vi "Test_Multiple Class_Multiple State.vi"() -> ()   [LabVIEW 2021]
uses:
  Commander/Commander.lvclass
  C:/Program Files (x86)/Hyper State Machine Framework/SSW_Hyper_State_Machine.lvlibp/State_Machine_Class/Main_State_Machine/Hyper_State_Machine.lvclass
  C:/Program Files (x86)/Hyper State Machine Framework/SSW_Hyper_State_Machine.lvlibp/State_Interface/State_Interface.lvclass
  Common_State/Common_State.lvclass
  Image_Acquisition/Image_Acquisition.lvclass
  Motion_Control/Motion_Control.lvclass
  Data_Logging/Data_Logging.lvclass
  DIO/DIO.lvclass
  C:/Program Files (x86)/Hyper State Machine Framework/SSW_Hyper_State_Machine.lvlibp/State_Machine_Class/State_Machine_Module.llb/State Machine.ctl
  C:/Program Files (x86)/Hyper State Machine Framework/SSW_Hyper_State_Machine.lvlibp/State_Machine_Class/State_Machine_Module.llb/Lock_Unlock.ctl
  C:/Program Files (x86)/Hyper State Machine Framework/SSW_Hyper_State_Machine.lvlibp/State_Machine_Class/State_Machine_Module.llb/Iterval.ctl
  C:/Program Files (x86)/Hyper State Machine Framework/SSW_Hyper_State_Machine.lvlibp/State_Machine_Class/State_Machine_Module.llb/Time_Out.ctl
  <vilib>/numeric/Random Number (Range) DBL.vi
  <vilib>/Utility/High Resolution Relative Seconds.vi
  C:/Program Files (x86)/Hyper State Machine Framework/SSW_Hyper_State_Machine.lvlibp
panel:
  out "Activate":bool
  out "Lamp":bool
  out "Current_Pos":dbl caption="mm"
  in  "EMO":bool
  out "Product ID":string
  in  "Activate_Code(Blank for 30 min Trial)":string="ROeInPkJ3DxAXwEgzbbW2XA0t1jaS1URlS9jikesQMED6VfU"
  out "Heart_Rate":bool
  out "Heart rate(s)":dbl format="%#_6p"
  out "Execute rate(Hz)":dbl format="%#_6p"
  out "Base Class_Time_Act":bool
  out "Base Class_Elapsed Time(s)":dbl format="%#_6p"
  out "Base Class":bool=TRUE
  out "Base Class_Remaining(s)":dbl format="%#_6p"
  out "Base Class Progress":dbl(slide) scale=0.0..10.0
  in  "Base Class":dbl=10.0 max=1000.0 format="%#_13p"
  out "Base Class":string
  out "Base Class_Active":bool
  in  "Action Manager":T1(ring)
  out "Common":bool=TRUE
  out "Common_State":string
  out "Common_Time_Act":bool
  out "Common_Elapsed Time(s)":dbl format="%#_6p"
  out "Common_State Progress":dbl(slide) scale=0.0..5.0
  in  "Common_State_Interval":dbl=5.0 max=1000.0 format="%#_13p"
  out "Common_State_Active":bool
  out "Common_State_Remaining(s)":dbl format="%#_6p"
  out "Data Logging Progress":dbl(slide) scale=0.0..3.0
  out "DIO Progress":dbl(slide) scale=0.0..0.01
  out "Motion Control Progress":dbl(slide) scale=0.0..0.5
  out "Image Acquisition Progress":dbl(slide) scale=0.0..0.25
  out "Commander Progress":dbl(slide)=-1.0 scale=0.0..1.0
  out "Data_Logging":bool=TRUE
  out "Data Logging":string
  out "Data_Logging_Time_Act":bool
  out "Data_Logging_Elapsed Time(s)":dbl format="%#_6p"
  out "DIO":bool=TRUE
  out "DIO":string
  out "DIO_Time_Act":bool
  out "DIO_Elapsed Time(s)":dbl format="%#_6p"
  out "Motion_Control":bool=TRUE
  out "Motion_Control":string
  out "Motion_Control_Time_Act":bool
  out "Motion_Control_Elapsed Time(s)":dbl format="%#_6p"
  in  "Data Logging":dbl=3.0 max=1000.0 format="%#_13p"
  out "Data Logging_Active":bool
  out "Data Logging_Remaining(s)":dbl format="%#_6p"
  in  "DIO_Interval":dbl=0.01 max=1000.0 format="%#_13p"
  in  "Motion_Control_Interval":dbl=0.5 max=1000.0 format="%#_13p"
  out "Motion Control_Act":bool
  out "DIO_Act":bool
  out "DIO_Remaining(s)":dbl format="%#_6p"
  out "Motion_Control_Remaining(s)":dbl format="%#_6p"
  in  "Image Acquisition_Interval":dbl=0.25 max=1000.0 format="%#_13p"
  in  "Commander_Interval":dbl max=1000.0 format="%#_13p"
  in  "System_Wait_Time":dbl=0.025 format="%#_13p"
  out "Commander_Active":bool
  out "Image Acquisition_Act":bool
  out "Image Acquisition_Remaining(s)":dbl format="%#_6p"
  out "Commander_Remaining(s)":dbl format="%#_6p"
  out "Image Acquisition":bool=TRUE
  out "Image Acquisition":string
  out "Commander":bool=TRUE
  out "Image Acquisition_Time_Act":bool
  out "Image Acquisition_Elapsed Time(s)":dbl format="%#_6p"
  out "Commander":string
  out "State1_Time_Act":bool
  out "Commander_Elapsed Time(s)":dbl format="%#_6p"
  in  "Stop":bool
  # "Note : Each State is Waiting Until Commader State Finished on \"Interval_Delay\" and then Unlock"
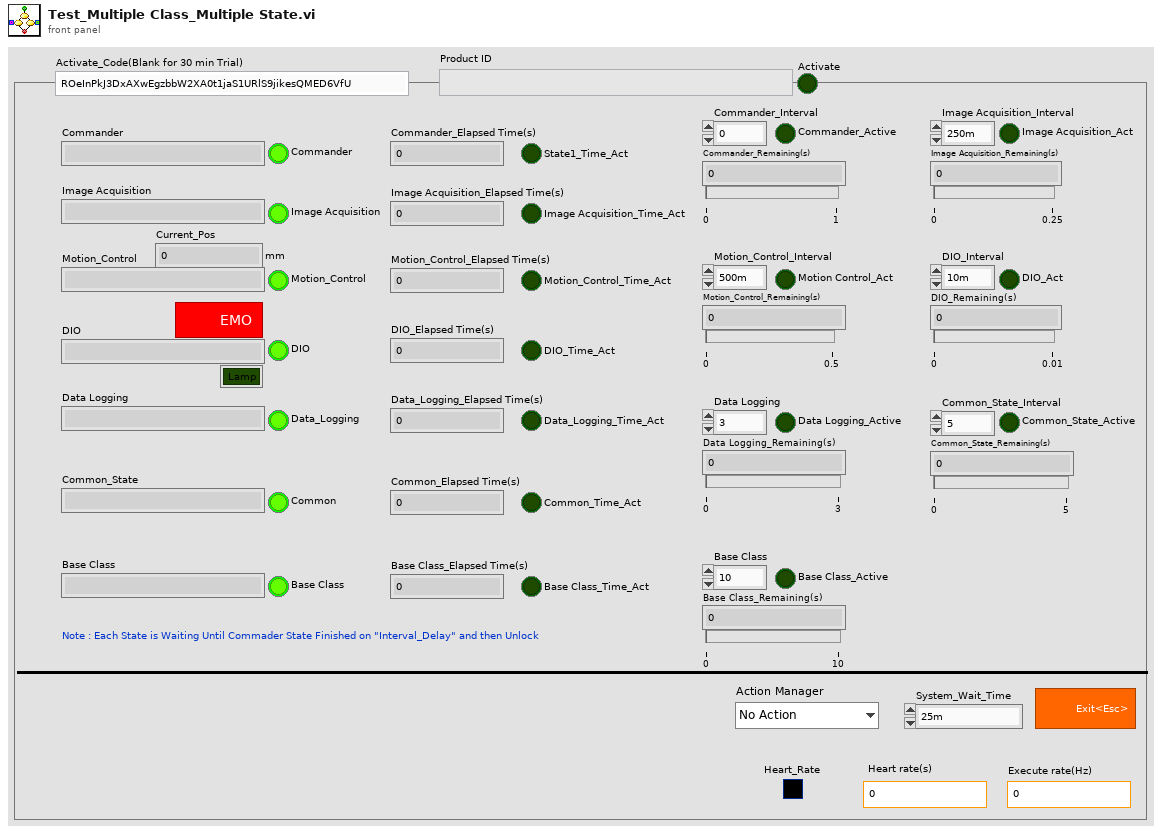
[diagram p1: front panel]
types:
  T1 = enum16{"No Action", "Init", "Lock", "Unlock", "Release"}
  T2 = typedef "SSW_Hyper_State_Machine.lvlibp/State Machine.ctl" = cluster{"Command":string, "Data":variant}
  T3 = typedef "SSW_Hyper_State_Machine.lvlibp/Time_Out.ctl" = cluster{"Enable(True)":bool, "Time Out_State Name":string, "Time Target (1s)":dbl, "Time Out_Reply Message_State":string}
  T4 = typedef "SSW_Hyper_State_Machine.lvlibp/Lock_Unlock.ctl" = cluster{"Action_Mode (Get)":enum16{"Set", "Get"}, "Action_Set (False)":bool, "State_In (Wait)":string}
  T5 = typedef "SSW_Hyper_State_Machine.lvlibp/Iterval.ctl" = cluster{"Delay(s)":dbl, "State (Interval_Delay)":string}
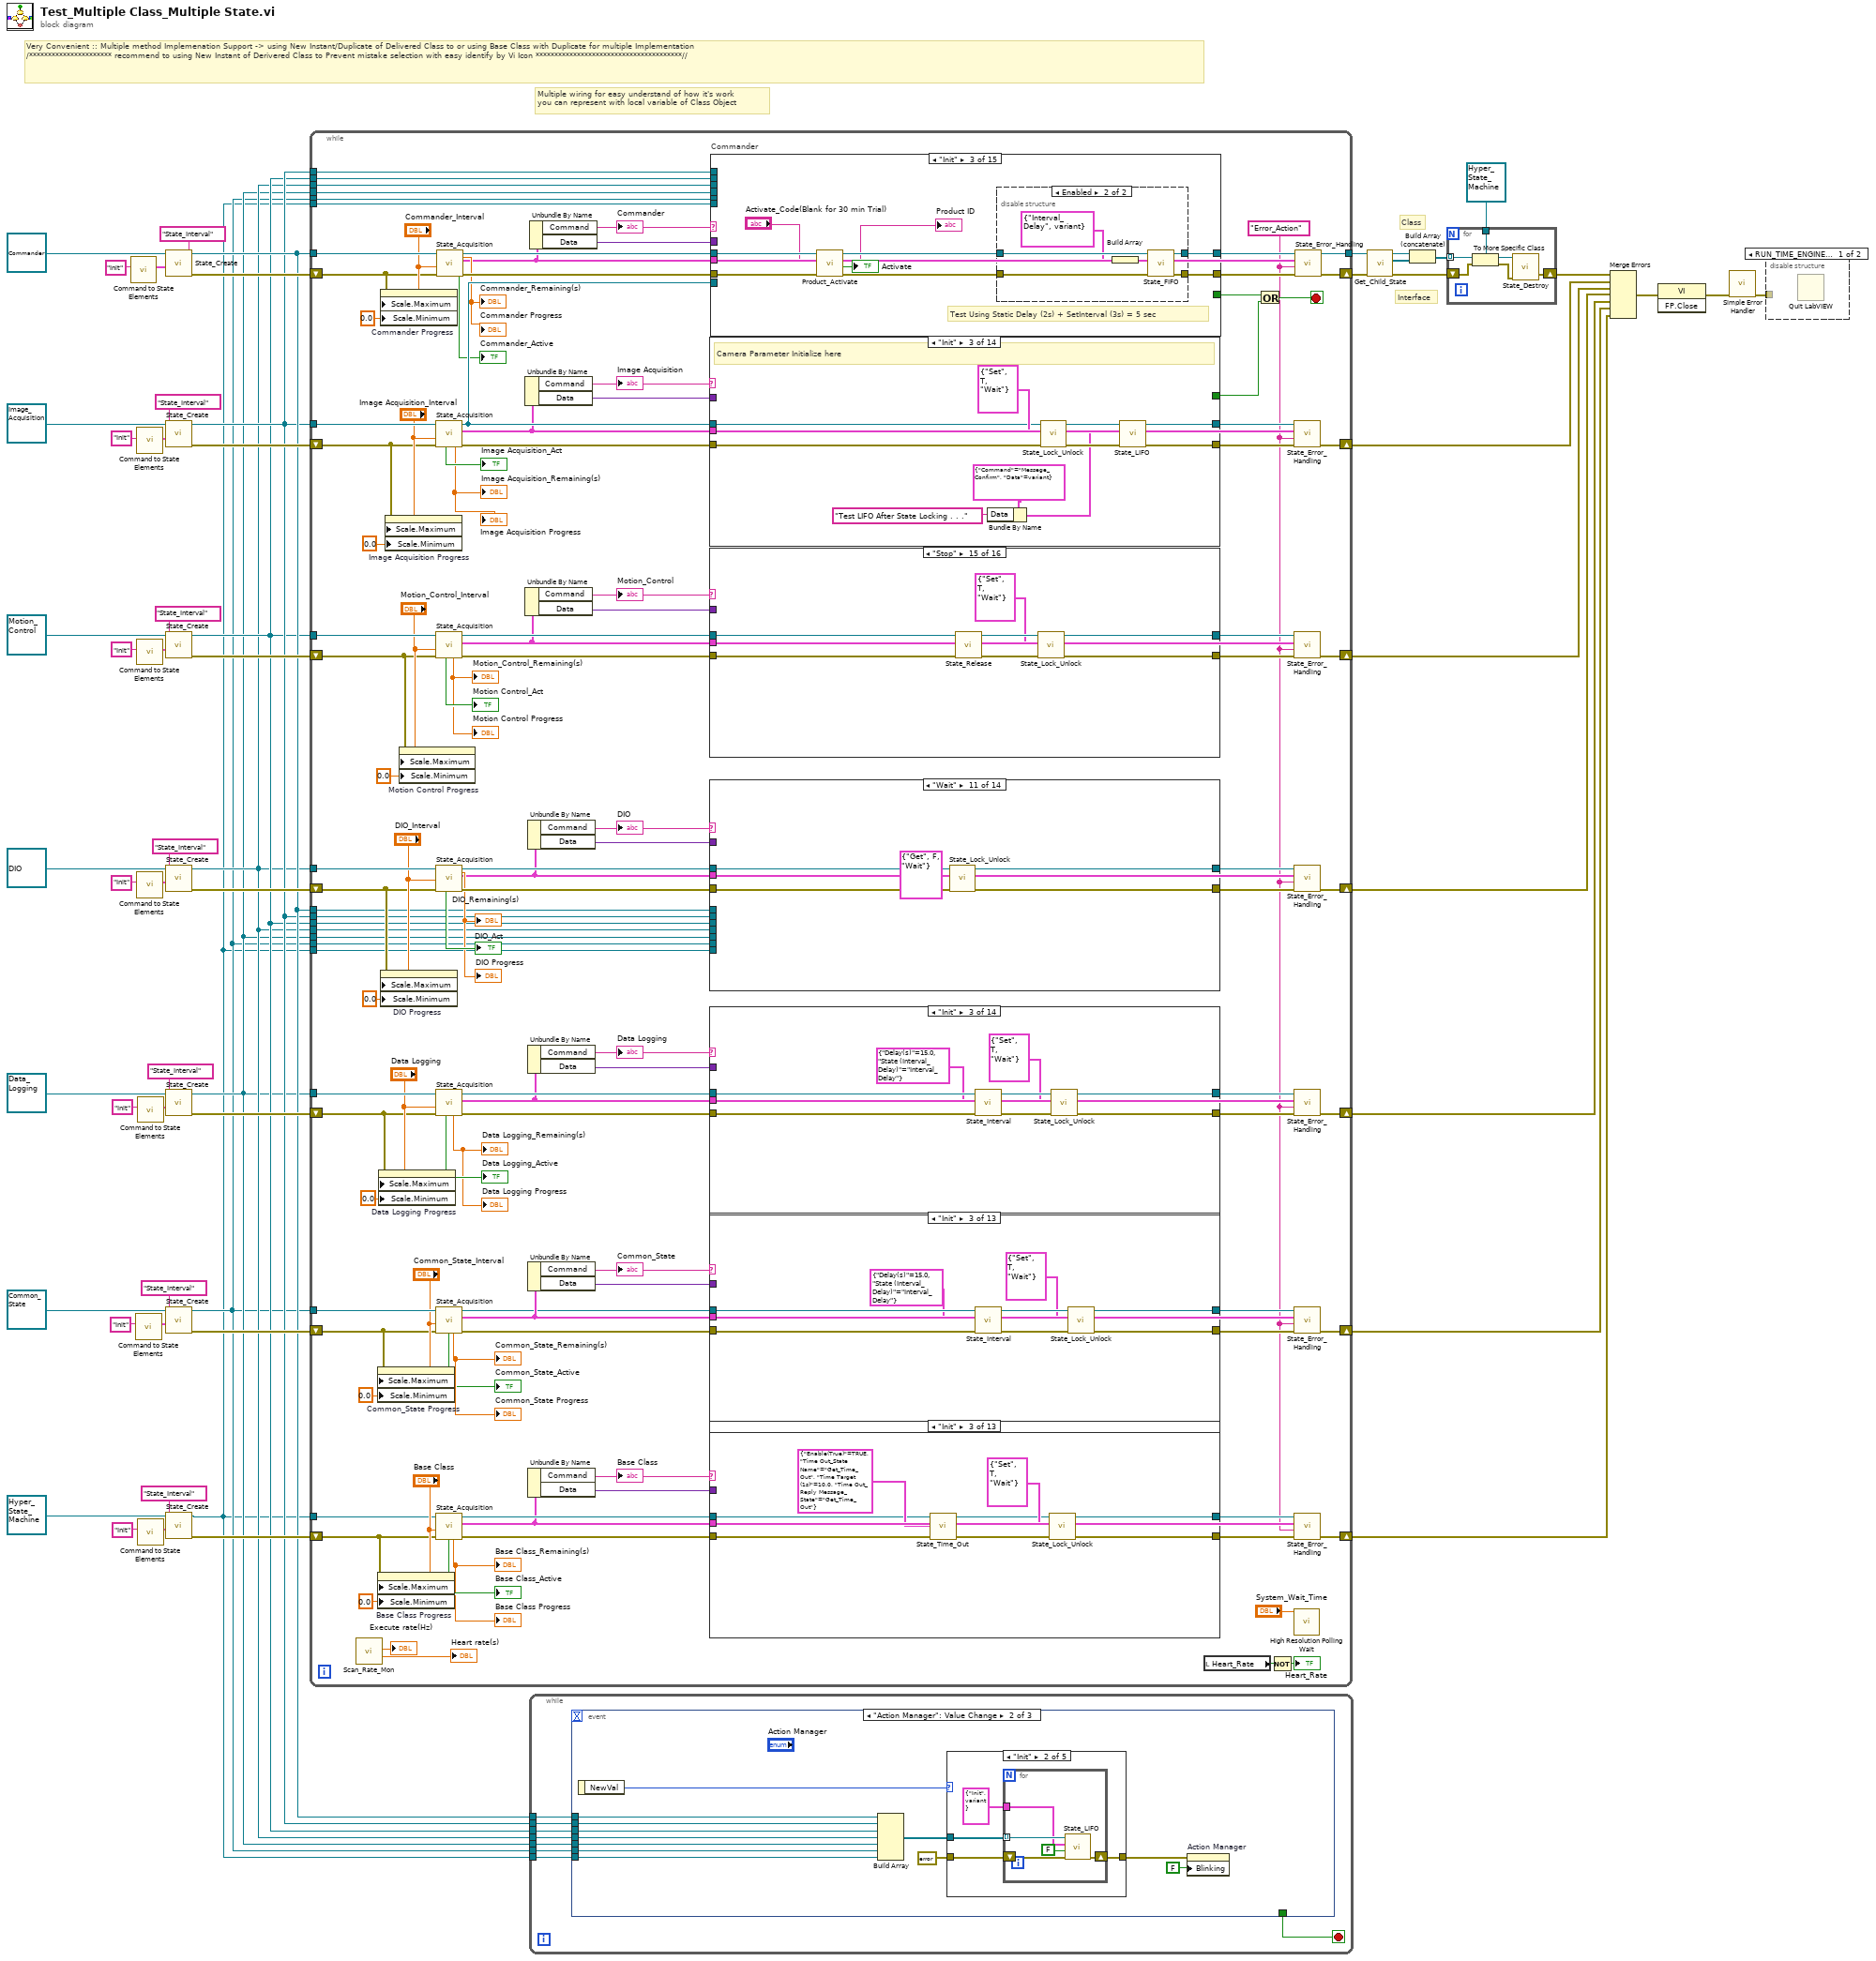
[diagram p0: block diagram]
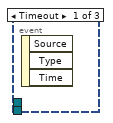
[diagram p3: hidden frame]
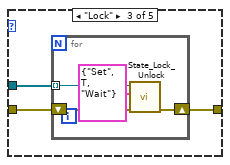
[diagram p5: hidden frame]
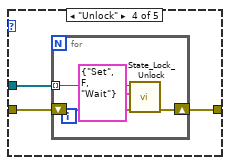
[diagram p6: hidden frame]
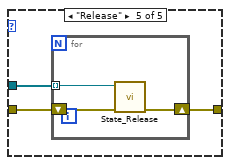
[diagram p7: hidden frame]
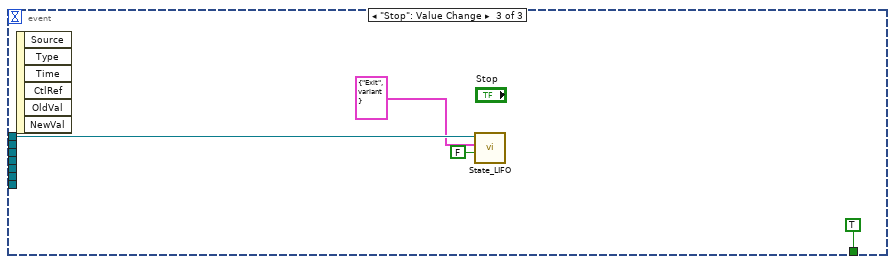
[diagram p8: hidden frame]
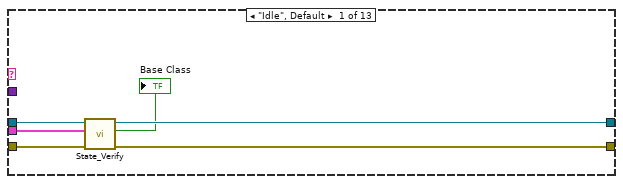
[diagram p9: hidden frame]
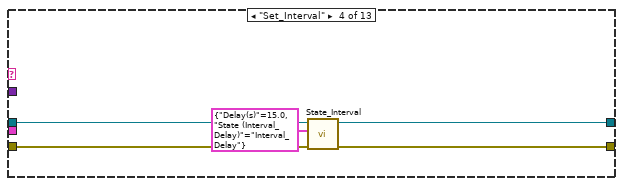
[diagram p11: hidden frame]
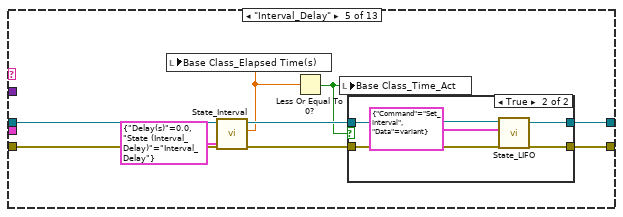
[diagram p12: hidden frame]
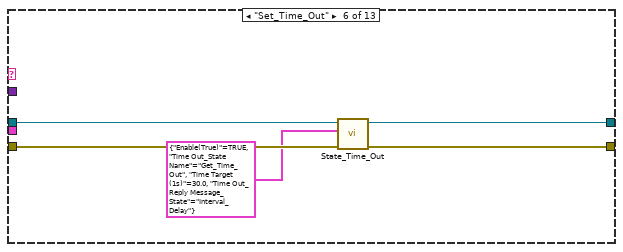
[diagram p14: hidden frame]
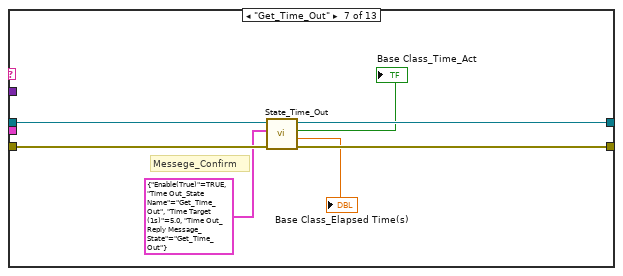
[diagram p15: hidden frame]
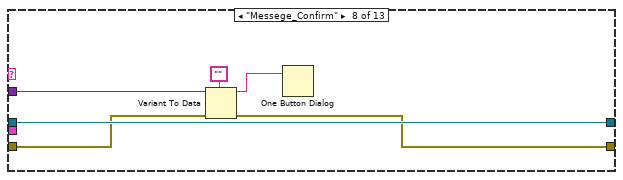
[diagram p16: hidden frame]
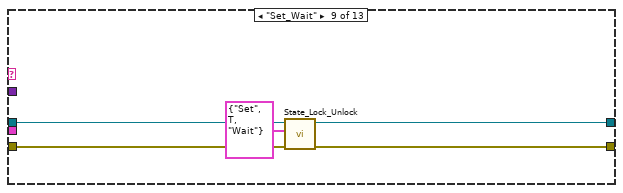
[diagram p17: hidden frame]
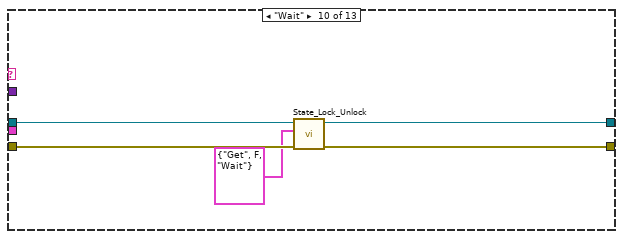
[diagram p18: hidden frame]
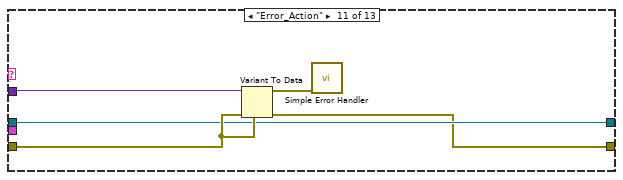
[diagram p19: hidden frame]
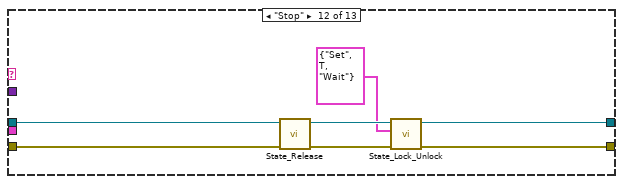
[diagram p20: hidden frame]
diagram:
  # "Interface"
  # "Class"
  # "Multiple wiring for easy understand of how it's work\nyou can represent with local variable of Class Object"
  # "Very Convenient :: Multiple method Implemenation Support -> using New Instant/Duplicate of Delivered Class to or using Base Class with Duplicate for multiple Implementation\n/********************** recommend to using New Instant of Derivered Class to Prevent mistake selection with easy identify by Vi Icon ***************************************//"
  n1 = call "Command to State Elements.vi"("Command"="Init") -> ("Command to State Elements"=w42:T2)  [unwired: 10 in]
  n2 = call "Command to State Elements.vi"("Command"="Init") -> ("Command to State Elements"=w34:T2)  [unwired: 10 in]
  n3 = call "Command to State Elements.vi"("Command"="Init") -> ("Command to State Elements"=w44:T2)  [unwired: 10 in]
  n4 = call "Command to State Elements.vi"("Command"="Init") -> ("Command to State Elements"=w40:T2)  [unwired: 10 in]
  n5 = call "Command to State Elements.vi"("Command"="Init") -> ("Command to State Elements"=w38:T2)  [unwired: 10 in]
  n6 = call "Command to State Elements.vi"("Command"="Init") -> ("Command to State Elements"=w36:T2)  [unwired: 10 in]
  n7 = call "Command to State Elements.vi"("Command"="Init") -> ("Command to State Elements"=w32:T2)  [unwired: 10 in]
  n8 = call-dynamic "State_Create.vi"("Init_State(Option)"=w42, "State_Interval_Name"="State_Interval" ("Core_Interval_Name(State_Interval)"), "State_Machine_Class in"=refnum<class "Commander.lvclass"> refnum ("Commander.lvclass")) -> ("error out"=w59:errorcluster, "State_Machine_Class out"=w24:refnum<class "Commander.lvclass">)  [unwired: 6 in, 1 out]
  n9 = call-dynamic "State_Create.vi"("Init_State(Option)"=w44, "State_Interval_Name"="State_Interval" ("Core_Interval_Name(State_Interval)"), "State_Machine_Class in"=refnum<class "Image_Acquisition.lvclass"> refnum ("Image_Acquisition.lvclass")) -> ("error out"=w58:errorcluster, "State_Machine_Class out"=w23:refnum<class "Image_Acquisition.lvclass">)  [unwired: 6 in, 1 out]
  n10 = call-dynamic "State_Create.vi"("Init_State(Option)"=w40, "State_Interval_Name"="State_Interval" ("Core_Interval_Name(State_Interval)"), "State_Machine_Class in"=refnum<class "Motion_Control.lvclass"> refnum ("Motion_Control.lvclass")) -> ("error out"=w53:errorcluster, "State_Machine_Class out"=w22:refnum<class "Motion_Control.lvclass">)  [unwired: 6 in, 1 out]
  n11 = call-dynamic "State_Create.vi"("Init_State(Option)"=w38, "State_Interval_Name"="State_Interval" ("Core_Interval_Name(State_Interval)"), "State_Machine_Class in"=refnum<class "DIO.lvclass"> refnum ("DIO.lvclass")) -> ("error out"=w52:errorcluster, "State_Machine_Class out"=w21:refnum<class "DIO.lvclass">)  [unwired: 6 in, 1 out]
  n12 = call-dynamic "State_Create.vi"("Init_State(Option)"=w36, "State_Interval_Name"="State_Interval" ("Core_Interval_Name(State_Interval)"), "State_Machine_Class in"=refnum<class "Data_Logging.lvclass"> refnum ("Data_Logging.lvclass")) -> ("error out"=w51:errorcluster, "State_Machine_Class out"=w20:refnum<class "Data_Logging.lvclass">)  [unwired: 6 in, 1 out]
  n13 = call-dynamic "State_Create.vi"("Init_State(Option)"=w34, "State_Interval_Name"="State_Interval" ("Core_Interval_Name(State_Interval)"), "State_Machine_Class in"=refnum<class "Common_State.lvclass"> refnum ("Common_State.lvclass")) -> ("error out"=w49:errorcluster, "State_Machine_Class out"=w19:refnum<class "Common_State.lvclass">)  [unwired: 6 in, 1 out]
  n14 = call-dynamic "State_Create.vi"("Init_State(Option)"=w32, "State_Interval_Name"="State_Interval" ("Core_Interval_Name(State_Interval)"), "State_Machine_Class in"=refnum<class "Hyper_State_Machine.lvclass"> refnum ("SSW_Hyper_State_Machine.lvlibp:Hyper_State_Machine.lvclass")) -> ("error out"=w46:errorcluster, "State_Machine_Class out"=w18:refnum<class "Hyper_State_Machine.lvclass">)  [unwired: 6 in, 1 out]
  n15 = while {
    tunnel: w24 -> [w166]
    shift-right: [w174] -> w16
    shift-left: w59 -> [w79]
    tunnel: [w173] -> w17
    tunnel: w23 -> [w169]
    shift-right: [w168] -> w9
    shift-left: w58 -> [w78]
    tunnel: w22 -> [w144]
    tunnel: w21 -> [w143]
    tunnel: w20 -> [w142]
    shift-right: [w141] -> w8
    shift-left: w53 -> [w77]
    shift-right: [w140] -> w7
    shift-left: w52 -> [w76]
    shift-right: [w139] -> w6
    shift-left: w51 -> [w75]
    tunnel: w19 -> [w118]
    shift-right: [w117] -> w5
    shift-left: w49 -> [w74]
    shift-right: [w87] -> w4
    shift-left: w46 -> [w73]
    tunnel: w18 -> [w91]
    tunnel: w23 -> [w72]
    tunnel: w22 -> [w71]
    tunnel: w21 -> [w70]
    tunnel: w20 -> [w69]
    tunnel: w19 -> [w68]
    tunnel: w18 -> [w67]
    tunnel: w24 -> [w66]
    tunnel: w23 -> [w65]
    tunnel: w22 -> [w64]
    tunnel: w21 -> [w63]
    tunnel: w20 -> [w62]
    tunnel: w19 -> [w61]
    tunnel: w18 -> [w60]
    stop <- w165 stop-if-true
    w86 = "Error_Action" ("State_Error_Handling")
    n16 = call "Scan_Rate_Mon.vi"() -> ("Heart rate(s)"=→"Heart rate(s)":dbl, "Execute rate(Hz)"=→"Execute rate(Hz)":dbl)
    n17 = property on="Common_State Progress" class="Slide (strict)"(error in=w74, "Scale.Maximum"="Common_State_Interval", "Scale.Minimum"=0.0 ("Scale.Range:Minimum")) -> ()  [unwired: 1 in, 2 out]
    n18 = property on="Base Class Progress" class="Slide (strict)"(error in=w73, "Scale.Maximum"="Base Class", "Scale.Minimum"=0.0 ("Scale.Range:Minimum")) -> ()  [unwired: 1 in, 2 out]
    n19 = property on="Data Logging Progress" class="Slide (strict)"(error in=w75, "Scale.Maximum"="Data Logging", "Scale.Minimum"=0.0 ("Scale.Range:Minimum")) -> ()  [unwired: 1 in, 2 out]
    n20 = property on="Commander Progress" class="Slide (strict)"(error in=w79, "Scale.Maximum"="Commander_Interval", "Scale.Minimum"=0.0 ("Scale.Range:Minimum")) -> ()  [unwired: 1 in, 2 out]
    n21 = property on="DIO Progress" class="Slide (strict)"(error in=w76, "Scale.Maximum"="DIO_Interval", "Scale.Minimum"=0.0 ("Scale.Range:Minimum")) -> ()  [unwired: 1 in, 2 out]
    n22 = property on="Image Acquisition Progress" class="Slide (strict)"(error in=w78, "Scale.Maximum"="Image Acquisition_Interval", "Scale.Minimum"=0.0 ("Scale.Range:Minimum")) -> ()  [unwired: 1 in, 2 out]
    n23 = property on="Motion Control Progress" class="Slide (strict)"(error in=w77, "Scale.Maximum"="Motion_Control_Interval", "Scale.Minimum"=0.0 ("Scale.Range:Minimum")) -> ()  [unwired: 1 in, 2 out]
    n24 = call-dynamic "State_Acquisition.vi"("error in (no error)"=w78, "State_Interval_Time(s)"="Image Acquisition_Interval", "Main_Machine_State_Class in"=w169) -> ("error out"=w172:errorcluster, "State"=w104:T2, "Main_Machine_State_Class out"=w167:refnum<class "Image_Acquisition.lvclass">, "Remaining(ms)"=→"Image Acquisition_Remaining(s)" →"Image Acquisition Progress":dbl, "Current_State_Active"=→"Image Acquisition_Act":bool)  [unwired: 2 in, 2 out]
    n25 = call-dynamic "State_Acquisition.vi"("error in (no error)"=w77, "State_Interval_Time(s)"="Motion_Control_Interval", "Main_Machine_State_Class in"=w144) -> ("error out"=w146:errorcluster, "State"=w103:T2, "Main_Machine_State_Class out"=w147:refnum<class "Motion_Control.lvclass">, "Remaining(ms)"=→"Motion_Control_Remaining(s)" →"Motion Control Progress":dbl, "Current_State_Active"=→"Motion Control_Act":bool)  [unwired: 2 in, 2 out]
    n26 = call-dynamic "State_Acquisition.vi"("error in (no error)"=w76, "State_Interval_Time(s)"="DIO_Interval", "Main_Machine_State_Class in"=w143) -> ("error out"=w153:errorcluster, "State"=w102:T2, "Main_Machine_State_Class out"=w154:refnum<class "DIO.lvclass">, "Remaining(ms)"=→"DIO_Remaining(s)" →"DIO Progress":dbl, "Current_State_Active"=→"DIO_Act":bool)  [unwired: 2 in, 2 out]
    n27 = call-dynamic "State_Acquisition.vi"("error in (no error)"=w75, "State_Interval_Time(s)"="Data Logging", "Main_Machine_State_Class in"=w142) -> ("error out"=w155:errorcluster, "State"=w101:T2, "Main_Machine_State_Class out"=w156:refnum<class "Data_Logging.lvclass">, "Remaining(ms)"=→"Data Logging_Remaining(s)" →"Data Logging Progress":dbl, "Current_State_Active"=→"Data Logging_Active":bool)  [unwired: 2 in, 2 out]
    n28 = call-dynamic "State_Acquisition.vi"("error in (no error)"=w74, "State_Interval_Time(s)"="Common_State_Interval", "Main_Machine_State_Class in"=w118) -> ("error out"=w120:errorcluster, "State"=w100:T2, "Main_Machine_State_Class out"=w85:refnum<class "Common_State.lvclass">, "Remaining(ms)"=→"Common_State_Remaining(s)" →"Common_State Progress":dbl, "Current_State_Active"=→"Common_State_Active":bool)  [unwired: 2 in, 2 out]
    n29 = call-dynamic "State_Acquisition.vi"("error in (no error)"=w73, "State_Interval_Time(s)"="Base Class", "Main_Machine_State_Class in"=w91) -> ("error out"=w92:errorcluster, "State"=w89:T2, "Main_Machine_State_Class out"=w93:refnum<class "Hyper_State_Machine.lvclass">, "Remaining(ms)"=→"Base Class_Remaining(s)" →"Base Class Progress":dbl, "Current_State_Active"=→"Base Class_Active":bool)  [unwired: 2 in, 2 out]
    n30 = call-dynamic "State_Acquisition.vi"("error in (no error)"=w79, "State_Interval_Time(s)"="Commander_Interval", "Main_Machine_State_Class in"=w166) -> ("error out"=w176:errorcluster, "State"=w105:T2, "Main_Machine_State_Class out"=w177:refnum<class "Commander.lvclass">, "Remaining(ms)"=→"Commander_Remaining(s)" →"Commander Progress":dbl, "Current_State_Active"=→"Commander_Active":bool)  [unwired: 2 in, 2 out]
    n31 = Unbundle By Name(w104) -> ("Command"=w170:string, "Data"=w171:variant)
    "Image Acquisition" <- w170
    n32 = Unbundle By Name(w103) -> ("Command"=w133:string, "Data"=w159:variant)
    "Motion_Control" <- w133
    n33 = Unbundle By Name(w102) -> ("Command"=w134:string, "Data"=w158:variant)
    "DIO" <- w134
    n34 = Unbundle By Name(w101) -> ("Command"=w135:string, "Data"=w157:variant)
    "Data Logging" <- w135
    n35 = Unbundle By Name(w100) -> ("Command"=w114:string, "Data"=w119:variant)
    "Common_State" <- w114
    n36 = Unbundle By Name(w89) -> ("Command"=w97:string, "Data"=w94:variant)
    "Base Class" <- w97
    n37 = Unbundle By Name(w105) -> ("Command"=w180:string, "Data"=w179:variant)
    "Commander" <- w180
    n38 = case shown="\"Init\"" w170 {
      selector: w170 -> [_ _ _ w666 _ _ _ _ _ _ _ _ _ _]
      tunnel: w171 -> [_ _ _ _ _ _ _ _ w720 _ _ w734 _ _]
      tunnel: w167 -> [w652 w654 w663 w671 w676 w689 w707 w714 w718 w725 w730 w731 w742 w747]
      tunnel: w172 -> [w651 w653 w662 w670 w675 w688 w706 w713 w717 w724 w729 w733 w741 w746]
      tunnel: [w645 w654 w660 w669 w674 w684 w705 w712 w718 w723 w728 w731 w737 w745] -> w161
      tunnel: [w644 w653 w658 w668 w673 w683 w704 w711 w716 w722 w727 w732 w736 w744] -> w160
      tunnel: w104 -> [w650 _ _ _ _ _ _ _ _ _ _ _ _ _]
      tunnel: [_ _ _ _ _ _ _ _ _ _ _ _ _ TRUE] -> w164
      frame "Idle", Default {
        n39 = call-dynamic "State_Verify.vi"("error in (no error)"=w651, "State(Idle)"=w650, "State_Machine_Class in"=w652) -> ("error out"=w647:errorcluster, "Active"=→"Image Acquisition":bool, "State_Machine_Class out"=w648:refnum<class "Image_Acquisition.lvclass">)  [unwired: 6 in]
        n40 = Build Array(T2 {"Command"="Image_Acquisition", "Data"=variant} ("State")) -> (w643:T2[])
        n41 = call-dynamic "State_FIFO.vi"("error in (no error)"=w647, "State Machine[]"=w643, "State_Machine_Class in"=w648) -> ("error out"=w644:errorcluster, "State_Machine_Class out"=w645:refnum<class "Image_Acquisition.lvclass">)  [unwired: 7 in]
      }
      frame "State_Interval" {
      }
      frame "Init" {
        # "Camera Parameter Initialize here"
        n42 = Bundle By Name(cluster=T2 {"Command"="Messege_Confirm", "Data"=variant} ("State Machine"), "Data"="Test LIFO After State Locking . . .") -> (w656:T2)
        n43 = call-dynamic "State_Lock_Unlock.vi"("error in (no error)"=w662, "Parameter"=T4 {"Action_Mode (Get)"=enum."Set", "Action_Set (False)"=TRUE, "State_In (Wait)"="Wait"}, "State_Machine_Class in"=w663) -> ("error out"=w659:errorcluster, "State_Machine_Class out"=w661:refnum<class "Image_Acquisition.lvclass">)  [unwired: 6 in, 1 out]
        n44 = call-dynamic "State_LIFO.vi"("error in (no error)"=w659, "State Machine"=w656, "State_Machine_Class in"=w661) -> ("error out"=w658:errorcluster, "State_Machine_Class out"=w660:refnum<class "Image_Acquisition.lvclass">)  [unwired: 7 in]
      }
      frame "Image_Acquisition" {
        (unwired) T5 {"Delay(s)"=5.0, "State (Interval_Delay)"="Image_Acquisition"} ("Parameter")
        # "Simple handling with specify name"
        # "Dynamic handling Name for Waiting Demo"
        # "Image Acquisition Function Here"
        n45 = Bundle By Name(cluster=T5 {"Delay(s)"=5.0, "State (Interval_Delay)"=""} ("Parameter"), "State (Interval_Delay)"=w666) -> (w665:T5)
        n46 = call-dynamic "State_Interval.vi"("error in (no error)"=w670, "Parameter"=w665, "State_Machine_Class in"=w671) -> ("error out"=w668:errorcluster, "State_Machine_Class out"=w669:refnum<class "Image_Acquisition.lvclass">)  [unwired: 6 in, 1 out]
      }
      frame "Set_Interval" {
        n47 = call-dynamic "State_Interval.vi"("error in (no error)"=w675, "Parameter"=T5 {"Delay(s)"=15.0, "State (Interval_Delay)"="Interval_Delay"}, "State_Machine_Class in"=w676) -> ("error out"=w673:errorcluster, "State_Machine_Class out"=w674:refnum<class "Image_Acquisition.lvclass">)  [unwired: 6 in, 1 out]
      }
      frame "Interval_Delay" {
        n48 = call-dynamic "State_Interval.vi"("error in (no error)"=w688, "Parameter"=T5 {"Delay(s)"=0.0, "State (Interval_Delay)"="Interval_Delay"}, "State_Machine_Class in"=w689) -> ("error out"=w685:errorcluster, "Elapsed Time(s)"=w682:dbl, "State_Machine_Class out"=w686:refnum<class "Image_Acquisition.lvclass">)  [unwired: 6 in]
        "Image Acquisition_Elapsed Time(s)" <- w682
        n49 = Build Array(T2 {"Command"="Interval_Delay", "Data"=variant} ("State"), T2 {"Command"="Image_Acquisition", "Data"=variant} ("State")) -> (w678:T2[])
        n50 = Less Or Equal To 0?(x=w682) -> (x <= 0?=w687:bool)
        n51 = Reverse 1D Array(array=w678) -> (reversed array=w677:T2[])
        n52 = case shown="True" w687 {
          tunnel: w686 -> [w691 w696]
          tunnel: w685 -> [w690 w695]
          tunnel: [w691 w694] -> w684
          tunnel: [w690 w693] -> w683
          tunnel: w677 -> [_ w692]
          frame False {
          }
          frame True {
            n53 = for {
              shift-right: [w699] -> w694
              shift-left: w696 -> [w701]
              shift-right: [w698] -> w693
              shift-left: w695 -> [w700]
              tunnel: w692 -> [w697] mode=indexing
              n54 = call-dynamic "State_LIFO.vi"("error in (no error)"=w700, "State Machine"=w697, "State_Machine_Class in"=w701) -> ("error out"=w698:errorcluster, "State_Machine_Class out"=w699:refnum<class "Image_Acquisition.lvclass">)  [unwired: 7 in]
            }
          }
        }
        n55 = local write "Image Acquisition_Time_Act"(w687) -> ()
      }
      frame "Set_Time_Out" {
        n56 = call-dynamic "State_Time_Out.vi"("error in (no error)"=w706, "Parameter"=T3 {"Enable(True)"=TRUE, "Time Out_State Name"="Get_Time_Out", "Time Target (1s)"=30.0, "Time Out_Reply Message_State"="Messege_Confirm"}, "State_Machine_Class in"=w707) -> ("error out"=w704:errorcluster, "Timeout"=w703:bool, "State_Machine_Class out"=w705:refnum<class "Image_Acquisition.lvclass">)  [unwired: 5 in, 1 out]
        n57 = local write "Image Acquisition_Time_Act"(w703) -> ()
      }
      frame "Get_Time_Out" {
        # "Messege_Confirm"
        n58 = call-dynamic "State_Time_Out.vi"("error in (no error)"=w713, "Parameter"=T3 {"Enable(True)"=TRUE, "Time Out_State Name"="Get_Time_Out", "Time Target (1s)"=0.0, "Time Out_Reply Message_State"="Messege_Confirm"}, "State_Machine_Class in"=w714) -> ("error out"=w711:errorcluster, "Remaining Time (s)"=w710:dbl, "Timeout"=→"Image Acquisition_Time_Act":bool, "State_Machine_Class out"=w712:refnum<class "Image_Acquisition.lvclass">)  [unwired: 5 in]
        n59 = local write "Image Acquisition_Elapsed Time(s)"(w710) -> ()
      }
      frame "Messege_Confirm" {
        n60 = Variant To Data(error in=w717, type="", Variant=w720) -> (data=w715:string, error out=w716:errorcluster)
        n61 = One Button Dialog(message=w715) -> ()  [unwired: 1 in, 1 out]
      }
      frame "Set_Wait" {
        n62 = call-dynamic "State_Lock_Unlock.vi"("error in (no error)"=w724, "Parameter"=T4 {"Action_Mode (Get)"=enum."Set", "Action_Set (False)"=TRUE, "State_In (Wait)"="Wait"}, "State_Machine_Class in"=w725) -> ("error out"=w722:errorcluster, "State_Machine_Class out"=w723:refnum<class "Image_Acquisition.lvclass">)  [unwired: 6 in, 1 out]
      }
      frame "Wait" {
        n63 = call-dynamic "State_Lock_Unlock.vi"("error in (no error)"=w729, "Parameter"=T4 {"Action_Mode (Get)"=enum."Get", "Action_Set (False)"=FALSE, "State_In (Wait)"="Wait"}, "State_Machine_Class in"=w730) -> ("error out"=w727:errorcluster, "State_Machine_Class out"=w728:refnum<class "Image_Acquisition.lvclass">)  [unwired: 6 in, 1 out]
      }
      frame "Error_Action" {
        n64 = Variant To Data(error in=w733, type=w733, Variant=w734) -> (data=w735:errorcluster, error out=w732:errorcluster)
        n65 = call <vilib>:"Simple Error Handler.vi"("error in (no error)"=w735) -> ()  [unwired: 4 in, 5 out]
      }
      frame "Stop" {
        n66 = call-dynamic "State_Release.vi"("error in (no error)"=w741, "State_Machine_Class in"=w742) -> ("error out"=w739:errorcluster, "State_Machine_Class out"=w740:refnum<class "Image_Acquisition.lvclass">)  [unwired: 8 in]
        n67 = call-dynamic "State_Lock_Unlock.vi"("error in (no error)"=w739, "Parameter"=T4 {"Action_Mode (Get)"=enum."Set", "Action_Set (False)"=TRUE, "State_In (Wait)"="Wait"}, "State_Machine_Class in"=w740) -> ("error out"=w736:errorcluster, "State_Machine_Class out"=w737:refnum<class "Image_Acquisition.lvclass">)  [unwired: 6 in, 1 out]
      }
      frame "Exit" {
        n68 = call-dynamic "State_Release.vi"("error in (no error)"=w746, "State_Machine_Class in"=w747) -> ("error out"=w744:errorcluster, "State_Machine_Class out"=w745:refnum<class "Image_Acquisition.lvclass">)  [unwired: 8 in]
      }
    }
    n69 = case shown="\"Stop\"" w133 {
      tunnel: w159 -> [_ _ _ _ _ _ _ _ _ _ w616 _ _ w629 _ _]
      tunnel: w147 -> [w552 w554 w560 w568 w573 w576 w581 w590 w603 w610 w614 w621 w626 w630 w638 w642]
      tunnel: w146 -> [w551 w553 w558 w567 w572 w575 w580 w589 w602 w609 w613 w620 w625 w628 w637 w641]
      tunnel: [w545 w554 w562 w566 w571 w576 w579 w586 w601 w608 w614 w619 w624 w630 w634 w640] -> w148
      tunnel: [w544 w553 w561 w565 w570 w575 w578 w585 w600 w607 w612 w618 w623 w627 w633 w639] -> w145
      tunnel: w103 -> [w550 _ _ _ _ _ _ _ _ _ _ _ _ _ _ _]
      frame "Idle", Default {
        n70 = call-dynamic "State_Verify.vi"("error in (no error)"=w551, "State(Idle)"=w550, "State_Machine_Class in"=w552) -> ("error out"=w547:errorcluster, "Active"=→"Motion_Control":bool, "State_Machine_Class out"=w548:refnum<class "Motion_Control.lvclass">)  [unwired: 6 in]
        n71 = Build Array(T2 {"Command"="Motion_Move", "Data"=variant} ("State")) -> (w543:T2[])
        n72 = call-dynamic "State_FIFO.vi"("error in (no error)"=w547, "State Machine[]"=w543, "State_Machine_Class in"=w548) -> ("error out"=w544:errorcluster, "State_Machine_Class out"=w545:refnum<class "Motion_Control.lvclass">)  [unwired: 7 in]
      }
      frame "State_Interval" {
        # "Handling Motion I/O or Cirtical Task Here"
      }
      frame "Init" {
        # "Motion Parameter Initialize Here"
        n73 = Build Array(T2 {"Command"="Motion_Move", "Data"=variant} ("State")) -> (w555:T2[])
        n74 = call-dynamic "State_FIFO.vi"("error in (no error)"=w558, "State Machine[]"=w555, "State_Machine_Class in"=w560) -> ("error out"=w557:errorcluster, "State_Machine_Class out"=w559:refnum<class "Motion_Control.lvclass">)  [unwired: 7 in]
        n75 = call-dynamic "State_Lock_Unlock.vi"("error in (no error)"=w557, "Parameter"=T4 {"Action_Mode (Get)"=enum."Set", "Action_Set (False)"=TRUE, "State_In (Wait)"="Wait"}, "State_Machine_Class in"=w559) -> ("error out"=w561:errorcluster, "State_Machine_Class out"=w562:refnum<class "Motion_Control.lvclass">)  [unwired: 6 in, 1 out]
      }
      frame "Motion_Move" {
        # "Motion Move Command here"
        n76 = call-dynamic "State_LIFO.vi"("error in (no error)"=w567, "State Machine"=T2 {"Command"="Motion_Request_Pos", "Data"=variant} ("State"), "State_Machine_Class in"=w568) -> ("error out"=w565:errorcluster, "State_Machine_Class out"=w566:refnum<class "Motion_Control.lvclass">)  [unwired: 7 in]
      }
      frame "Motion_Request_Pos" {
        # "Motion Query Position Command here"
        n77 = call-dynamic "State_LIFO.vi"("error in (no error)"=w572, "State Machine"=T2 {"Command"="Motion_Get_Pos", "Data"=variant} ("State"), "State_Machine_Class in"=w573) -> ("error out"=w570:errorcluster, "State_Machine_Class out"=w571:refnum<class "Motion_Control.lvclass">)  [unwired: 7 in]
      }
      frame "Motion_Get_Pos" {
        # "Motion Move Command here"
        n78 = call-poly <vilib>:"Random Number (Range).vi"() -> ("number"=→"Current_Pos":dbl)  [unwired: 11 in]
      }
      frame "Set_Interval" {
        n79 = call-dynamic "State_Interval.vi"("error in (no error)"=w580, "Parameter"=T5 {"Delay(s)"=15.0, "State (Interval_Delay)"="Interval_Delay"}, "State_Machine_Class in"=w581) -> ("error out"=w578:errorcluster, "State_Machine_Class out"=w579:refnum<class "Motion_Control.lvclass">)  [unwired: 6 in, 1 out]
      }
      frame "Interval_Delay" {
        n80 = call-dynamic "State_Interval.vi"("error in (no error)"=w589, "Parameter"=T5 {"Delay(s)"=0.0, "State (Interval_Delay)"="Interval_Delay"}, "State_Machine_Class in"=w590) -> ("error out"=w587:errorcluster, "Elapsed Time(s)"=w584:dbl, "State_Machine_Class out"=w588:refnum<class "Motion_Control.lvclass">)  [unwired: 6 in]
        n81 = local write "Motion_Control_Elapsed Time(s)"(w584) -> ()
        n82 = Less Or Equal To 0?(x=w584) -> (x <= 0?=w583:bool)
        n83 = local write "Motion_Control_Time_Act"(w583) -> ()
        n84 = case shown="True" w583 {
          tunnel: w588 -> [w592 w598]
          tunnel: w587 -> [w591 w597]
          tunnel: [w592 w596] -> w586
          tunnel: [w591 w595] -> w585
          frame False {
          }
          frame True {
            n85 = call-dynamic "State_LIFO.vi"("error in (no error)"=w597, "State_Interval(Enable)"=FALSE, "State Machine"=T2 {"Command"="Set_Interval", "Data"=variant} ("State"), "State_Machine_Class in"=w598) -> ("error out"=w595:errorcluster, "State_Machine_Class out"=w596:refnum<class "Motion_Control.lvclass">)  [unwired: 6 in]
          }
        }
      }
      frame "Set_Time_Out" {
        n86 = call-dynamic "State_Time_Out.vi"("error in (no error)"=w602, "Parameter"=T3 {"Enable(True)"=TRUE, "Time Out_State Name"="Get_Time_Out", "Time Target (1s)"=30.0, "Time Out_Reply Message_State"="Messege_Confirm"}, "State_Machine_Class in"=w603) -> ("error out"=w600:errorcluster, "State_Machine_Class out"=w601:refnum<class "Motion_Control.lvclass">)  [unwired: 5 in, 2 out]
      }
      frame "Get_Time_Out" {
        # "Messege_Confirm"
        n87 = call-dynamic "State_Time_Out.vi"("error in (no error)"=w609, "Parameter"=T3 {"Enable(True)"=TRUE, "Time Out_State Name"="Get_Time_Out", "Time Target (1s)"=0.0, "Time Out_Reply Message_State"="Messege_Confirm"}, "State_Machine_Class in"=w610) -> ("error out"=w607:errorcluster, "Remaining Time (s)"=→"Motion_Control_Elapsed Time(s)":dbl, "Timeout"=→"Motion_Control_Time_Act":bool, "State_Machine_Class out"=w608:refnum<class "Motion_Control.lvclass">)  [unwired: 5 in]
      }
      frame "Messege_Confirm" {
        n88 = Variant To Data(error in=w613, type="", Variant=w616) -> (data=w611:string, error out=w612:errorcluster)
        n89 = One Button Dialog(message=w611) -> ()  [unwired: 1 in, 1 out]
      }
      frame "Set_Wait" {
        n90 = call-dynamic "State_Lock_Unlock.vi"("error in (no error)"=w620, "Parameter"=T4 {"Action_Mode (Get)"=enum."Set", "Action_Set (False)"=TRUE, "State_In (Wait)"="Wait"}, "State_Machine_Class in"=w621) -> ("error out"=w618:errorcluster, "State_Machine_Class out"=w619:refnum<class "Motion_Control.lvclass">)  [unwired: 6 in, 1 out]
      }
      frame "Wait" {
        n91 = call-dynamic "State_Lock_Unlock.vi"("error in (no error)"=w625, "Parameter"=T4 {"Action_Mode (Get)"=enum."Get", "Action_Set (False)"=FALSE, "State_In (Wait)"="Wait"}, "State_Machine_Class in"=w626) -> ("error out"=w623:errorcluster, "State_Machine_Class out"=w624:refnum<class "Motion_Control.lvclass">)  [unwired: 6 in, 1 out]
      }
      frame "Error_Action" {
        n92 = Variant To Data(error in=w628, type=w628, Variant=w629) -> (data=w631:errorcluster, error out=w627:errorcluster)
        n93 = call <vilib>:"Simple Error Handler.vi"("error in (no error)"=w631) -> ()  [unwired: 4 in, 5 out]
      }
      frame "Stop" {
        n94 = call-dynamic "State_Release.vi"("error in (no error)"=w637, "State_Machine_Class in"=w638) -> ("error out"=w635:errorcluster, "State_Machine_Class out"=w636:refnum<class "Motion_Control.lvclass">)  [unwired: 8 in]
        n95 = call-dynamic "State_Lock_Unlock.vi"("error in (no error)"=w635, "Parameter"=T4 {"Action_Mode (Get)"=enum."Set", "Action_Set (False)"=TRUE, "State_In (Wait)"="Wait"}, "State_Machine_Class in"=w636) -> ("error out"=w633:errorcluster, "State_Machine_Class out"=w634:refnum<class "Motion_Control.lvclass">)  [unwired: 6 in, 1 out]
      }
      frame "Exit" {
        n96 = call-dynamic "State_Release.vi"("error in (no error)"=w641, "State_Machine_Class in"=w642) -> ("error out"=w639:errorcluster, "State_Machine_Class out"=w640:refnum<class "Motion_Control.lvclass">)  [unwired: 8 in]
      }
    }
    n97 = case shown="\"Wait\"" w134 {
      tunnel: w158 -> [_ _ _ _ _ _ _ _ w513 _ _ w526 _ _]
      tunnel: w154 -> [w437 w447 w464 w479 w486 w491 w498 w504 w511 w518 w523 w524 w538 w542]
      tunnel: w153 -> [w436 w438 w463 w478 w485 w490 w497 w503 w510 w517 w522 w527 w537 w541]
      tunnel: [w431 w447 w467 w477 w481 w489 w496 w502 w511 w516 w521 w524 w534 w540] -> w152
      tunnel: [w430 w438 w466 w476 w480 w488 w495 w501 w509 w515 w520 w525 w531 w539] -> w151
      tunnel: w102 -> [w435 _ _ _ _ _ _ _ _ _ _ _ _ _]
      tunnel: w66 -> [_ w445 _ _ _ _ _ _ _ _ _ _ _ _]
      tunnel: w65 -> [_ w444 _ _ _ _ _ _ _ _ _ _ _ _]
      tunnel: w64 -> [_ w443 _ _ _ _ _ _ _ _ _ _ _ _]
      tunnel: w63 -> [_ w442 _ _ _ _ _ _ _ _ _ _ _ _]
      tunnel: w62 -> [_ w441 _ _ _ _ _ _ _ _ _ _ _ _]
      tunnel: w61 -> [_ w440 _ _ _ _ _ _ _ _ _ _ _ _]
      tunnel: w60 -> [_ w439 _ _ _ _ _ _ _ _ _ _ _ _]
      frame "Idle", Default {
        # "Able to activate at \"Stae_Interval\""
        n98 = call-dynamic "State_Verify.vi"("error in (no error)"=w436, "State(Idle)"=w435, "State_Machine_Class in"=w437) -> ("error out"=w432:errorcluster, "Active"=→"DIO":bool, "State_Machine_Class out"=w433:refnum<class "DIO.lvclass">)  [unwired: 6 in]
        n99 = Build Array(T2 {"Command"="Lamp_Blinking", "Data"=variant} ("State")) -> (w428:T2[])
        n100 = call-dynamic "State_FIFO.vi"("error in (no error)"=w432, "State Machine[]"=w428, "State_Machine_Class in"=w433) -> ("error out"=w430:errorcluster, "State_Machine_Class out"=w431:refnum<class "DIO.lvclass">)  [unwired: 7 in]
      }
      frame "State_Interval" {
        # "Able to assign to Even to handling"
        # "Simulation of Emergency Signal , Pree to try (Can not Override State Lock if in Active)"
        # "Simulation of Emergency Signal"
        # "Every Cycle Time DIO Get Data Here"
        n101 = case shown="True" "EMO" {
          tunnel: w445 -> [_ w457]
          tunnel: w444 -> [_ w456]
          tunnel: w443 -> [_ w455]
          tunnel: w442 -> [_ w454]
          tunnel: w441 -> [_ w453]
          tunnel: w440 -> [_ w452]
          tunnel: w439 -> [_ w451]
          tunnel: w438 -> [_ w448]
          frame False {
          }
          frame True {
            n102 = Build Array(w457, w456, w455, w454, w453, w452, w451) -> (w450:refnum<class "Hyper_State_Machine.lvclass">[])
            n103 = for {
              tunnel: w450 -> [w459] mode=indexing
              tunnel: T2 {"Command"="Stop", "Data"=variant} ("State") -> [w460]
              shift-right: [w462] -> _
              shift-left: w448 -> [w458]
              n104 = call-dynamic "State_LIFO.vi"("error in (no error)"=w458, "State_Interval(Enable)"=FALSE, "State Machine"=w460, "State_Machine_Class in"=w459) -> ("error out"=w462:errorcluster)  [unwired: 6 in, 1 out]
            }
          }
        }
      }
      frame "Init" {
        # "DIO Parameter Initialize here"
        n105 = disable-structure shown="Enabled" {
          disable-tunnel: [w472 w474] -> w467
          disable-tunnel: [w471 w473] -> w466
          disable-tunnel: w464 -> [w469 w474]
          disable-tunnel: w463 -> [w468 w473]
          frame Disabled {
            n106 = call-dynamic "State_Lock_Unlock.vi"("error in (no error)"=w468, "Parameter"=T4 {"Action_Mode (Get)"=enum."Set", "Action_Set (False)"=TRUE, "State_In (Wait)"="Wait"}, "State_Machine_Class in"=w469) -> ("error out"=w471:errorcluster, "State_Machine_Class out"=w472:refnum<class "DIO.lvclass">)  [unwired: 6 in, 1 out]
          }
          frame Enabled {
          }
        }
        "Lamp" <- FALSE ("Lamp")
      }
      frame "Set_Interval" {
        n107 = call-dynamic "State_Interval.vi"("error in (no error)"=w478, "Parameter"=T5 {"Delay(s)"=15.0, "State (Interval_Delay)"="Interval_Delay"}, "State_Machine_Class in"=w479) -> ("error out"=w476:errorcluster, "State_Machine_Class out"=w477:refnum<class "DIO.lvclass">)  [unwired: 6 in, 1 out]
      }
      frame "Interval_Delay" {
        n108 = call-dynamic "State_Interval.vi"("error in (no error)"=w485, "Parameter"=T5 {"Delay(s)"=0.0, "State (Interval_Delay)"="Interval_Delay"}, "State_Machine_Class in"=w486) -> ("error out"=w480:errorcluster, "Elapsed Time(s)"=w484:dbl, "State_Machine_Class out"=w481:refnum<class "DIO.lvclass">)  [unwired: 6 in]
        n109 = local write "DIO_Elapsed Time(s)"(w484) -> ()
        n110 = Less Or Equal To 0?(x=w484) -> (x <= 0?=w483:bool)
        n111 = local write "DIO_Time_Act"(w483) -> ()
      }
      frame "Set_Time_Out" {
        n112 = call-dynamic "State_Time_Out.vi"("error in (no error)"=w490, "Parameter"=T3 {"Enable(True)"=TRUE, "Time Out_State Name"="Get_Time_Out", "Time Target (1s)"=30.0, "Time Out_Reply Message_State"="Messege_Confirm"}, "State_Machine_Class in"=w491) -> ("error out"=w488:errorcluster, "State_Machine_Class out"=w489:refnum<class "DIO.lvclass">)  [unwired: 5 in, 2 out]
      }
      frame "Get_Time_Out" {
        # "Messege_Confirm"
        n113 = call-dynamic "State_Time_Out.vi"("error in (no error)"=w497, "Parameter"=T3 {"Enable(True)"=TRUE, "Time Out_State Name"="Get_Time_Out", "Time Target (1s)"=0.0, "Time Out_Reply Message_State"="Messege_Confirm"}, "State_Machine_Class in"=w498) -> ("error out"=w495:errorcluster, "Remaining Time (s)"=→"DIO_Elapsed Time(s)":dbl, "Timeout"=→"DIO_Time_Act":bool, "State_Machine_Class out"=w496:refnum<class "DIO.lvclass">)  [unwired: 5 in]
      }
      frame "Lamp_Blinking" {
        n114 = call-dynamic "State_Interval.vi"("error in (no error)"=w503, "Parameter"=T5 {"Delay(s)"=0.25, "State (Interval_Delay)"="Lamp_Blinking"}, "State_Machine_Class in"=w504) -> ("error out"=w501:errorcluster, "Elapsed Time(s)"=w499:dbl, "State_Machine_Class out"=w502:refnum<class "DIO.lvclass">)  [unwired: 6 in]
        n115 = Less Or Equal To 0?(x=w499) -> (x <= 0?=w500:bool)
        n116 = case shown="True" w500 {
          frame False {
          }
          frame True {
            n117 = local read "Lamp"() -> (w507:bool)
            n118 = Not(x=w507) -> (.not. x?=w506:bool)
            n119 = local write "Lamp"(w506) -> ()
          }
        }
      }
      frame "Messege_Confirm" {
        n120 = Variant To Data(error in=w510, type="", Variant=w513) -> (data=w508:string, error out=w509:errorcluster)
        n121 = One Button Dialog(message=w508) -> ()  [unwired: 1 in, 1 out]
      }
      frame "Set_Wait" {
        n122 = call-dynamic "State_Lock_Unlock.vi"("error in (no error)"=w517, "Parameter"=T4 {"Action_Mode (Get)"=enum."Set", "Action_Set (False)"=TRUE, "State_In (Wait)"="Wait"}, "State_Machine_Class in"=w518) -> ("error out"=w515:errorcluster, "State_Machine_Class out"=w516:refnum<class "DIO.lvclass">)  [unwired: 6 in, 1 out]
      }
      frame "Wait" {
        n123 = call-dynamic "State_Lock_Unlock.vi"("error in (no error)"=w522, "Parameter"=T4 {"Action_Mode (Get)"=enum."Get", "Action_Set (False)"=FALSE, "State_In (Wait)"="Wait"}, "State_Machine_Class in"=w523) -> ("error out"=w520:errorcluster, "State_Machine_Class out"=w521:refnum<class "DIO.lvclass">)  [unwired: 6 in, 1 out]
      }
      frame "Error_Action" {
        n124 = Variant To Data(error in=w527, type=w527, Variant=w526) -> (data=w528:errorcluster, error out=w525:errorcluster)
        n125 = call <vilib>:"Simple Error Handler.vi"("error in (no error)"=w528) -> ()  [unwired: 4 in, 5 out]
      }
      frame "Stop" {
        n126 = call-dynamic "State_Release.vi"("error in (no error)"=w537, "State_Machine_Class in"=w538) -> ("error out"=w535:errorcluster, "State_Machine_Class out"=w536:refnum<class "DIO.lvclass">)  [unwired: 8 in]
        n127 = call-dynamic "State_Lock_Unlock.vi"("error in (no error)"=w535, "Parameter"=T4 {"Action_Mode (Get)"=enum."Set", "Action_Set (False)"=TRUE, "State_In (Wait)"="Wait"}, "State_Machine_Class in"=w536) -> ("error out"=w532:errorcluster, "State_Machine_Class out"=w534:refnum<class "DIO.lvclass">)  [unwired: 6 in, 1 out]
        n128 = property on="Action Manager" class="Enum (strict)"(error in=w532, "Blinking"=TRUE) -> (error out=w531:errorcluster)  [unwired: 1 in, 1 out]
        n129 = One Button Dialog(message="All State is Locking !\nPlease Unlock With Action Manager to Release . . .") -> ()  [unwired: 1 in, 1 out]
      }
      frame "Exit" {
        n130 = call-dynamic "State_Release.vi"("error in (no error)"=w541, "State_Machine_Class in"=w542) -> ("error out"=w539:errorcluster, "State_Machine_Class out"=w540:refnum<class "DIO.lvclass">)  [unwired: 8 in]
      }
    }
    n131 = case shown="\"Init\"" w135 {
      tunnel: w157 -> [_ _ _ _ _ _ _ _ w401 _ _ w414 _ _]
      tunnel: w156 -> [w349 w351 w359 w361 w366 w375 w388 w395 w399 w406 w411 w413 w423 w427]
      tunnel: w155 -> [w348 w350 w358 w360 w365 w374 w387 w394 w398 w405 w410 w415 w422 w426]
      tunnel: [w346 w351 w355 w361 w364 w371 w386 w393 w399 w404 w409 w413 w418 w425] -> w150
      tunnel: [w345 w350 w354 w360 w363 w370 w385 w392 w397 w403 w408 w412 w417 w424] -> w149
      tunnel: w101 -> [w347 _ _ _ _ _ _ _ _ _ _ _ _ _]
      frame "Idle", Default {
        n132 = call-dynamic "State_Verify.vi"("error in (no error)"=w348, "State(Idle)"=w347, "State_Machine_Class in"=w349) -> ("error out"=w345:errorcluster, "Active"=→"Data_Logging":bool, "State_Machine_Class out"=w346:refnum<class "Data_Logging.lvclass">)  [unwired: 6 in]
      }
      frame "State_Interval" {
        # "Files Monitering or Cirtical Task Handling Here"
      }
      frame "Init" {
        n133 = call-dynamic "State_Interval.vi"("error in (no error)"=w358, "Parameter"=T5 {"Delay(s)"=15.0, "State (Interval_Delay)"="Interval_Delay"}, "State_Machine_Class in"=w359) -> ("error out"=w353:errorcluster, "State_Machine_Class out"=w356:refnum<class "Data_Logging.lvclass">)  [unwired: 6 in, 1 out]
        n134 = call-dynamic "State_Lock_Unlock.vi"("error in (no error)"=w353, "Parameter"=T4 {"Action_Mode (Get)"=enum."Set", "Action_Set (False)"=TRUE, "State_In (Wait)"="Wait"}, "State_Machine_Class in"=w356) -> ("error out"=w354:errorcluster, "State_Machine_Class out"=w355:refnum<class "Data_Logging.lvclass">)  [unwired: 6 in, 1 out]
      }
      frame "Data_Logging" {
        # "Save Data Files Here"
      }
      frame "Set_Interval" {
        n135 = call-dynamic "State_Interval.vi"("error in (no error)"=w365, "Parameter"=T5 {"Delay(s)"=15.0, "State (Interval_Delay)"="Interval_Delay"}, "State_Machine_Class in"=w366) -> ("error out"=w363:errorcluster, "State_Machine_Class out"=w364:refnum<class "Data_Logging.lvclass">)  [unwired: 6 in, 1 out]
      }
      frame "Interval_Delay" {
        n136 = call-dynamic "State_Interval.vi"("error in (no error)"=w374, "Parameter"=T5 {"Delay(s)"=0.0, "State (Interval_Delay)"="Interval_Delay"}, "State_Machine_Class in"=w375) -> ("error out"=w372:errorcluster, "Elapsed Time(s)"=w369:dbl, "State_Machine_Class out"=w373:refnum<class "Data_Logging.lvclass">)  [unwired: 6 in]
        n137 = local write "Data_Logging_Elapsed Time(s)"(w369) -> ()
        n138 = Less Or Equal To 0?(x=w369) -> (x <= 0?=w368:bool)
        n139 = local write "Data_Logging_Time_Act"(w368) -> ()
        n140 = case shown="True" w368 {
          tunnel: w373 -> [w377 w383]
          tunnel: w372 -> [w376 w382]
          tunnel: [w377 w381] -> w371
          tunnel: [w376 w380] -> w370
          frame False {
          }
          frame True {
            n141 = call-dynamic "State_LIFO.vi"("error in (no error)"=w382, "State_Interval(Enable)"=FALSE, "State Machine"=T2 {"Command"="Set_Interval", "Data"=variant} ("State"), "State_Machine_Class in"=w383) -> ("error out"=w380:errorcluster, "State_Machine_Class out"=w381:refnum<class "Data_Logging.lvclass">)  [unwired: 6 in]
          }
        }
      }
      frame "Set_Time_Out" {
        n142 = call-dynamic "State_Time_Out.vi"("error in (no error)"=w387, "Parameter"=T3 {"Enable(True)"=TRUE, "Time Out_State Name"="Get_Time_Out", "Time Target (1s)"=30.0, "Time Out_Reply Message_State"="Interval_Delay"}, "State_Machine_Class in"=w388) -> ("error out"=w385:errorcluster, "State_Machine_Class out"=w386:refnum<class "Data_Logging.lvclass">)  [unwired: 5 in, 2 out]
      }
      frame "Get_Time_Out" {
        # "Messege_Confirm"
        n143 = call-dynamic "State_Time_Out.vi"("error in (no error)"=w394, "Parameter"=T3 {"Enable(True)"=TRUE, "Time Out_State Name"="Get_Time_Out", "Time Target (1s)"=0.0, "Time Out_Reply Message_State"="Messege_Confirm"}, "State_Machine_Class in"=w395) -> ("error out"=w392:errorcluster, "Remaining Time (s)"=→"Data_Logging_Elapsed Time(s)":dbl, "Timeout"=→"Data_Logging_Time_Act":bool, "State_Machine_Class out"=w393:refnum<class "Data_Logging.lvclass">)  [unwired: 5 in]
      }
      frame "Messege_Confirm" {
        n144 = Variant To Data(error in=w398, type="", Variant=w401) -> (data=w396:string, error out=w397:errorcluster)
        n145 = One Button Dialog(message=w396) -> ()  [unwired: 1 in, 1 out]
      }
      frame "Set_Wait" {
        n146 = call-dynamic "State_Lock_Unlock.vi"("error in (no error)"=w405, "Parameter"=T4 {"Action_Mode (Get)"=enum."Set", "Action_Set (False)"=TRUE, "State_In (Wait)"="Wait"}, "State_Machine_Class in"=w406) -> ("error out"=w403:errorcluster, "State_Machine_Class out"=w404:refnum<class "Data_Logging.lvclass">)  [unwired: 6 in, 1 out]
      }
      frame "Wait" {
        n147 = call-dynamic "State_Lock_Unlock.vi"("error in (no error)"=w410, "Parameter"=T4 {"Action_Mode (Get)"=enum."Get", "Action_Set (False)"=TRUE, "State_In (Wait)"="Wait"}, "State_Machine_Class in"=w411) -> ("error out"=w408:errorcluster, "State_Machine_Class out"=w409:refnum<class "Data_Logging.lvclass">)  [unwired: 6 in, 1 out]
      }
      frame "Error_Action" {
        n148 = Variant To Data(error in=w415, type=w415, Variant=w414) -> (data=w416:errorcluster, error out=w412:errorcluster)
        n149 = call <vilib>:"Simple Error Handler.vi"("error in (no error)"=w416) -> ()  [unwired: 4 in, 5 out]
      }
      frame "Stop" {
        n150 = call-dynamic "State_Release.vi"("error in (no error)"=w422, "State_Machine_Class in"=w423) -> ("error out"=w420:errorcluster, "State_Machine_Class out"=w421:refnum<class "Data_Logging.lvclass">)  [unwired: 8 in]
        n151 = call-dynamic "State_Lock_Unlock.vi"("error in (no error)"=w420, "Parameter"=T4 {"Action_Mode (Get)"=enum."Set", "Action_Set (False)"=TRUE, "State_In (Wait)"="Wait"}, "State_Machine_Class in"=w421) -> ("error out"=w417:errorcluster, "State_Machine_Class out"=w418:refnum<class "Data_Logging.lvclass">)  [unwired: 6 in, 1 out]
      }
      frame "Exit" {
        n152 = call-dynamic "State_Release.vi"("error in (no error)"=w426, "State_Machine_Class in"=w427) -> ("error out"=w424:errorcluster, "State_Machine_Class out"=w425:refnum<class "Data_Logging.lvclass">)  [unwired: 8 in]
      }
    }
    n153 = case shown="\"Init\"" w114 {
      tunnel: w119 -> [_ _ _ _ _ _ _ w317 _ _ w331 _ _]
      tunnel: w85 -> [w267 w269 w277 w282 w283 w304 w311 w315 w322 w327 w329 w339 w343]
      tunnel: w120 -> [w266 w268 w276 w281 w291 w303 w310 w314 w321 w326 w330 w338 w342]
      tunnel: [w264 w269 w271 w280 w288 w302 w309 w315 w320 w325 w329 w334 w341] -> w121
      tunnel: [w263 w268 w270 w279 w287 w301 w308 w313 w319 w324 w328 w333 w340] -> w122
      tunnel: w100 -> [w265 _ _ _ _ _ _ _ _ _ _ _ _]
      frame "Idle", Default {
        n154 = call-dynamic "State_Verify.vi"("error in (no error)"=w266, "State(Idle)"=w265, "State_Machine_Class in"=w267) -> ("error out"=w263:errorcluster, "Active"=→"Common":bool, "State_Machine_Class out"=w264:refnum<class "Common_State.lvclass">)  [unwired: 6 in]
      }
      frame "State_Interval" {
        # "Cirtical Task Handling Here"
      }
      frame "Init" {
        n155 = call-dynamic "State_Interval.vi"("error in (no error)"=w276, "Parameter"=T5 {"Delay(s)"=15.0, "State (Interval_Delay)"="Interval_Delay"}, "State_Machine_Class in"=w277) -> ("error out"=w273:errorcluster, "State_Machine_Class out"=w274:refnum<class "Common_State.lvclass">)  [unwired: 6 in, 1 out]
        n156 = call-dynamic "State_Lock_Unlock.vi"("error in (no error)"=w273, "Parameter"=T4 {"Action_Mode (Get)"=enum."Set", "Action_Set (False)"=TRUE, "State_In (Wait)"="Wait"}, "State_Machine_Class in"=w274) -> ("error out"=w270:errorcluster, "State_Machine_Class out"=w271:refnum<class "Common_State.lvclass">)  [unwired: 6 in, 1 out]
      }
      frame "Set_Interval" {
        n157 = call-dynamic "State_Interval.vi"("error in (no error)"=w281, "Parameter"=T5 {"Delay(s)"=15.0, "State (Interval_Delay)"="Interval_Delay"}, "State_Machine_Class in"=w282) -> ("error out"=w279:errorcluster, "State_Machine_Class out"=w280:refnum<class "Common_State.lvclass">)  [unwired: 6 in, 1 out]
      }
      frame "Interval_Delay" {
        n158 = call-dynamic "State_Interval.vi"("error in (no error)"=w291, "Parameter"=T5 {"Delay(s)"=5.0, "State (Interval_Delay)"="Interval_Delay"}, "State_Machine_Class in"=w283) -> ("error out"=w289:errorcluster, "Elapsed Time(s)"=w286:dbl, "State_Machine_Class out"=w290:refnum<class "Common_State.lvclass">)  [unwired: 6 in]
        n159 = local write "Common_Elapsed Time(s)"(w286) -> ()
        n160 = Less Or Equal To 0?(x=w286) -> (x <= 0?=w285:bool)
        n161 = local write "Common_Time_Act"(w285) -> ()
        n162 = case shown="True" w285 {
          tunnel: w290 -> [w293 w299]
          tunnel: w289 -> [w292 w298]
          tunnel: [w293 w297] -> w288
          tunnel: [w292 w296] -> w287
          frame False {
          }
          frame True {
            n163 = call-dynamic "State_LIFO.vi"("error in (no error)"=w298, "State_Interval(Enable)"=FALSE, "State Machine"=T2 {"Command"="Interval_Delay", "Data"=variant} ("State"), "State_Machine_Class in"=w299) -> ("error out"=w296:errorcluster, "State_Machine_Class out"=w297:refnum<class "Common_State.lvclass">)  [unwired: 6 in]
          }
        }
      }
      frame "Set_Time_Out" {
        n164 = call-dynamic "State_Time_Out.vi"("error in (no error)"=w303, "Parameter"=T3 {"Enable(True)"=TRUE, "Time Out_State Name"="Get_Time_Out", "Time Target (1s)"=30.0, "Time Out_Reply Message_State"="Interval_Delay"}, "State_Machine_Class in"=w304) -> ("error out"=w301:errorcluster, "State_Machine_Class out"=w302:refnum<class "Common_State.lvclass">)  [unwired: 5 in, 2 out]
      }
      frame "Get_Time_Out" {
        # "Messege_Confirm"
        # "Messege_Confirm"
        n165 = call-dynamic "State_Time_Out.vi"("error in (no error)"=w310, "Parameter"=T3 {"Enable(True)"=TRUE, "Time Out_State Name"="Get_Time_Out", "Time Target (1s)"=0.0, "Time Out_Reply Message_State"="Set_Interval"}, "State_Machine_Class in"=w311) -> ("error out"=w308:errorcluster, "Remaining Time (s)"=→"Common_Elapsed Time(s)":dbl, "Timeout"=→"Common_Time_Act":bool, "State_Machine_Class out"=w309:refnum<class "Common_State.lvclass">)  [unwired: 5 in]
      }
      frame "Messege_Confirm" {
        n166 = Variant To Data(error in=w314, type="", Variant=w317) -> (data=w312:string, error out=w313:errorcluster)
        n167 = One Button Dialog(message=w312) -> ()  [unwired: 1 in, 1 out]
      }
      frame "Set_Wait" {
        n168 = call-dynamic "State_Lock_Unlock.vi"("error in (no error)"=w321, "Parameter"=T4 {"Action_Mode (Get)"=enum."Set", "Action_Set (False)"=TRUE, "State_In (Wait)"="Wait"}, "State_Machine_Class in"=w322) -> ("error out"=w319:errorcluster, "State_Machine_Class out"=w320:refnum<class "Common_State.lvclass">)  [unwired: 6 in, 1 out]
      }
      frame "Wait" {
        n169 = call-dynamic "State_Lock_Unlock.vi"("error in (no error)"=w326, "Parameter"=T4 {"Action_Mode (Get)"=enum."Get", "Action_Set (False)"=FALSE, "State_In (Wait)"="Wait"}, "State_Machine_Class in"=w327) -> ("error out"=w324:errorcluster, "State_Machine_Class out"=w325:refnum<class "Common_State.lvclass">)  [unwired: 6 in, 1 out]
      }
      frame "Error_Action" {
        n170 = Variant To Data(error in=w330, type=w330, Variant=w331) -> (data=w332:errorcluster, error out=w328:errorcluster)
        n171 = call <vilib>:"Simple Error Handler.vi"("error in (no error)"=w332) -> ()  [unwired: 4 in, 5 out]
      }
      frame "Stop" {
        n172 = call-dynamic "State_Release.vi"("error in (no error)"=w338, "State_Machine_Class in"=w339) -> ("error out"=w336:errorcluster, "State_Machine_Class out"=w337:refnum<class "Common_State.lvclass">)  [unwired: 8 in]
        n173 = call-dynamic "State_Lock_Unlock.vi"("error in (no error)"=w336, "Parameter"=T4 {"Action_Mode (Get)"=enum."Set", "Action_Set (False)"=TRUE, "State_In (Wait)"="Wait"}, "State_Machine_Class in"=w337) -> ("error out"=w333:errorcluster, "State_Machine_Class out"=w334:refnum<class "Common_State.lvclass">)  [unwired: 6 in, 1 out]
      }
      frame "Exit" {
        n174 = call-dynamic "State_Release.vi"("error in (no error)"=w342, "State_Machine_Class in"=w343) -> ("error out"=w340:errorcluster, "State_Machine_Class out"=w341:refnum<class "Common_State.lvclass">)  [unwired: 8 in]
      }
    }
    n175 = case shown="\"Init\"" w97 {
      tunnel: w94 -> [_ _ _ _ _ _ _ w235 _ _ w249 _ _]
      tunnel: w93 -> [w186 w188 w192 w201 w210 w222 w229 w233 w240 w245 w247 w257 w261]
      tunnel: w92 -> [w185 w187 w190 w200 w209 w221 w228 w232 w239 w244 w248 w256 w260]
      tunnel: [w183 w188 w196 w199 w206 w220 w227 w233 w238 w243 w247 w252 w259] -> w90
      tunnel: [w182 w187 w195 w198 w205 w219 w226 w231 w237 w242 w246 w251 w258] -> w88
      tunnel: w89 -> [w184 _ _ _ _ _ _ _ _ _ _ _ _]
      frame "Idle", Default {
        n176 = call-dynamic "State_Verify.vi"("error in (no error)"=w185, "State(Idle)"=w184, "State_Machine_Class in"=w186) -> ("error out"=w182:errorcluster, "Active"=→"Base Class":bool, "State_Machine_Class out"=w183:refnum<class "Hyper_State_Machine.lvclass">)  [unwired: 6 in]
      }
      frame "State_Interval" {
        # "Cirtical Task Handling Here"
      }
      frame "Init" {
        n177 = call-dynamic "State_Time_Out.vi"("error in (no error)"=w190, "Parameter"=T3 {"Enable(True)"=TRUE, "Time Out_State Name"="Get_Time_Out", "Time Target (1s)"=10.0, "Time Out_Reply Message_State"="Get_Time_Out"}, "State_Machine_Class in"=w192) -> ("error out"=w189:errorcluster, "State_Machine_Class out"=w191:refnum<class "Hyper_State_Machine.lvclass">)  [unwired: 5 in, 2 out]
        n178 = call-dynamic "State_Lock_Unlock.vi"("error in (no error)"=w189, "Parameter"=T4 {"Action_Mode (Get)"=enum."Set", "Action_Set (False)"=TRUE, "State_In (Wait)"="Wait"}, "State_Machine_Class in"=w191) -> ("error out"=w195:errorcluster, "State_Machine_Class out"=w196:refnum<class "Hyper_State_Machine.lvclass">)  [unwired: 6 in, 1 out]
      }
      frame "Set_Interval" {
        n179 = call-dynamic "State_Interval.vi"("error in (no error)"=w200, "Parameter"=T5 {"Delay(s)"=15.0, "State (Interval_Delay)"="Interval_Delay"}, "State_Machine_Class in"=w201) -> ("error out"=w198:errorcluster, "State_Machine_Class out"=w199:refnum<class "Hyper_State_Machine.lvclass">)  [unwired: 6 in, 1 out]
      }
      frame "Interval_Delay" {
        n180 = call-dynamic "State_Interval.vi"("error in (no error)"=w209, "Parameter"=T5 {"Delay(s)"=0.0, "State (Interval_Delay)"="Interval_Delay"}, "State_Machine_Class in"=w210) -> ("error out"=w207:errorcluster, "Elapsed Time(s)"=w204:dbl, "State_Machine_Class out"=w208:refnum<class "Hyper_State_Machine.lvclass">)  [unwired: 6 in]
        n181 = local write "Base Class_Elapsed Time(s)"(w204) -> ()
        n182 = Less Or Equal To 0?(x=w204) -> (x <= 0?=w203:bool)
        n183 = local write "Base Class_Time_Act"(w203) -> ()
        n184 = case shown="True" w203 {
          tunnel: w208 -> [w212 w217]
          tunnel: w207 -> [w211 w216]
          tunnel: [w212 w215] -> w206
          tunnel: [w211 w214] -> w205
          frame False {
          }
          frame True {
            n185 = call-dynamic "State_LIFO.vi"("error in (no error)"=w216, "State Machine"=T2 {"Command"="Set_Interval", "Data"=variant} ("State"), "State_Machine_Class in"=w217) -> ("error out"=w214:errorcluster, "State_Machine_Class out"=w215:refnum<class "Hyper_State_Machine.lvclass">)  [unwired: 7 in]
          }
        }
      }
      frame "Set_Time_Out" {
        n186 = call-dynamic "State_Time_Out.vi"("error in (no error)"=w221, "Parameter"=T3 {"Enable(True)"=TRUE, "Time Out_State Name"="Get_Time_Out", "Time Target (1s)"=30.0, "Time Out_Reply Message_State"="Interval_Delay"}, "State_Machine_Class in"=w222) -> ("error out"=w219:errorcluster, "State_Machine_Class out"=w220:refnum<class "Hyper_State_Machine.lvclass">)  [unwired: 5 in, 2 out]
      }
      frame "Get_Time_Out" {
        # "Messege_Confirm"
        n187 = call-dynamic "State_Time_Out.vi"("error in (no error)"=w228, "Parameter"=T3 {"Enable(True)"=TRUE, "Time Out_State Name"="Get_Time_Out", "Time Target (1s)"=5.0, "Time Out_Reply Message_State"="Get_Time_Out"}, "State_Machine_Class in"=w229) -> ("error out"=w226:errorcluster, "Remaining Time (s)"=→"Base Class_Elapsed Time(s)":dbl, "Timeout"=→"Base Class_Time_Act":bool, "State_Machine_Class out"=w227:refnum<class "Hyper_State_Machine.lvclass">)  [unwired: 5 in]
      }
      frame "Messege_Confirm" {
        n188 = Variant To Data(error in=w232, type="", Variant=w235) -> (data=w230:string, error out=w231:errorcluster)
        n189 = One Button Dialog(message=w230) -> ()  [unwired: 1 in, 1 out]
      }
      frame "Set_Wait" {
        n190 = call-dynamic "State_Lock_Unlock.vi"("error in (no error)"=w239, "Parameter"=T4 {"Action_Mode (Get)"=enum."Set", "Action_Set (False)"=TRUE, "State_In (Wait)"="Wait"}, "State_Machine_Class in"=w240) -> ("error out"=w237:errorcluster, "State_Machine_Class out"=w238:refnum<class "Hyper_State_Machine.lvclass">)  [unwired: 6 in, 1 out]
      }
      frame "Wait" {
        n191 = call-dynamic "State_Lock_Unlock.vi"("error in (no error)"=w244, "Parameter"=T4 {"Action_Mode (Get)"=enum."Get", "Action_Set (False)"=FALSE, "State_In (Wait)"="Wait"}, "State_Machine_Class in"=w245) -> ("error out"=w242:errorcluster, "State_Machine_Class out"=w243:refnum<class "Hyper_State_Machine.lvclass">)  [unwired: 6 in, 1 out]
      }
      frame "Error_Action" {
        n192 = Variant To Data(error in=w248, type=w248, Variant=w249) -> (data=w250:errorcluster, error out=w246:errorcluster)
        n193 = call <vilib>:"Simple Error Handler.vi"("error in (no error)"=w250) -> ()  [unwired: 4 in, 5 out]
      }
      frame "Stop" {
        n194 = call-dynamic "State_Release.vi"("error in (no error)"=w256, "State_Machine_Class in"=w257) -> ("error out"=w254:errorcluster, "State_Machine_Class out"=w255:refnum<class "Hyper_State_Machine.lvclass">)  [unwired: 8 in]
        n195 = call-dynamic "State_Lock_Unlock.vi"("error in (no error)"=w254, "Parameter"=T4 {"Action_Mode (Get)"=enum."Set", "Action_Set (False)"=TRUE, "State_In (Wait)"="Wait"}, "State_Machine_Class in"=w255) -> ("error out"=w251:errorcluster, "State_Machine_Class out"=w252:refnum<class "Hyper_State_Machine.lvclass">)  [unwired: 6 in, 1 out]
      }
      frame "Exit" {
        n196 = call-dynamic "State_Release.vi"("error in (no error)"=w260, "State_Machine_Class in"=w261) -> ("error out"=w258:errorcluster, "State_Machine_Class out"=w259:refnum<class "Hyper_State_Machine.lvclass">)  [unwired: 8 in]
      }
    }
    n197 = case "Commander" shown="\"Init\"" w180 {
      tunnel: w179 -> [_ _ _ _ _ _ _ w818 w826 _ _ _ w852 _ _]
      tunnel: w177 -> [w753 w755 w762 w780 w790 w805 w812 w816 w822 w836 w844 w848 w853 w860 w865]
      tunnel: w176 -> [w751 w754 w761 w779 w789 w804 w811 w815 w825 _ w843 w847 w849 w859 w864]
      tunnel: [w750 w755 w764 w778 w785 w803 w810 w816 w822 w836 w842 w846 w853 w856 w863] -> w106
      tunnel: [w749 w754 w763 w777 w784 w802 w809 w814 w821 w835 w841 w845 w850 w855 w862] -> w175
      tunnel: [_ _ _ _ _ _ _ _ _ _ _ _ _ _ TRUE] -> w178
      tunnel: w105 -> [w752 _ _ _ w781 _ _ _ _ _ _ _ _ _ _]
      tunnel: w167 -> [_ _ _ _ _ _ _ _ _ _ _ _ _ _ _]
      tunnel: w72 -> [_ _ _ _ _ _ _ _ _ w833 _ _ _ _ _]
      tunnel: w71 -> [_ _ _ _ _ _ _ _ _ w832 _ _ _ _ _]
      tunnel: w70 -> [_ _ _ _ _ _ _ _ _ w831 _ _ _ _ _]
      tunnel: w69 -> [_ _ _ _ _ _ _ _ _ w830 _ _ _ _ _]
      tunnel: w68 -> [_ _ _ _ _ _ _ _ _ w829 _ _ _ _ _]
      tunnel: w67 -> [_ _ _ _ _ _ _ _ _ w828 _ _ _ _ _]
      frame "Idle", Default {
        n198 = call-dynamic "State_Verify.vi"("error in (no error)"=w751, "State(Idle)"=w752, "State_Machine_Class in"=w753) -> ("error out"=w749:errorcluster, "Active"=→"Commander":bool, "State_Machine_Class out"=w750:refnum<class "Commander.lvclass">)  [unwired: 6 in]
      }
      frame "State_Interval" {
      }
      frame "Init" {
        # "Test Using Static Delay (2s) + SetInterval (3s) = 5 sec"
        n199 = call-dynamic "Product_Activate.vi"("error in (no error)"=w761, "Activate Code"="Activate_Code(Blank for 30 min Trial)", "Commander in"=w762) -> ("error out"=w759:errorcluster, "Activate"=→"Activate":bool, "Product ID"=→"Product ID":string, "Commander out"=w760:refnum<class "Commander.lvclass">)  [unwired: 5 in]
        n200 = disable-structure shown="Enabled" {
          disable-tunnel: [w769 w774] -> w764
          disable-tunnel: [w768 w773] -> w763
          disable-tunnel: w760 -> [w766 w775]
          disable-tunnel: w759 -> [w765 w772]
          frame Disabled {
            n201 = call-dynamic "State_Interval.vi"("error in (no error)"=w765, "Parameter"=T5 {"Delay(s)"=5.0, "State (Interval_Delay)"="Interval_Delay"}, "State_Machine_Class in"=w766) -> ("error out"=w768:errorcluster, "State_Machine_Class out"=w769:refnum<class "Commander.lvclass">)  [unwired: 6 in, 1 out]
          }
          frame Enabled {
            n202 = Build Array(T2 {"Command"="Interval_Delay", "Data"=variant} ("State")) -> (w770:T2[])
            n203 = call-dynamic "State_FIFO.vi"("error in (no error)"=w772, "State Machine[]"=w770, "State_Machine_Class in"=w775) -> ("error out"=w773:errorcluster, "State_Machine_Class out"=w774:refnum<class "Commander.lvclass">)  [unwired: 7 in]
          }
        }
      }
      frame "Set_Interval" {
        n204 = call-dynamic "State_Interval.vi"("error in (no error)"=w779, "Parameter"=T5 {"Delay(s)"=3.0, "State (Interval_Delay)"="Interval_Delay"}, "State_Machine_Class in"=w780) -> ("error out"=w777:errorcluster, "State_Machine_Class out"=w778:refnum<class "Commander.lvclass">)  [unwired: 6 in, 1 out]
      }
      frame "Interval_Delay" {
        n205 = call-dynamic "State_Interval.vi"("error in (no error)"=w789, "Parameter"=T5 {"Delay(s)"=5.0, "State (Interval_Delay)"="Interval_Delay"}, "State_Machine_Class in"=w790) -> ("error out"=w786:errorcluster, "Elapsed Time(s)"=w783:dbl, "State_Machine_Class out"=w787:refnum<class "Commander.lvclass">)  [unwired: 6 in]
        "Commander_Elapsed Time(s)" <- w783
        n206 = Less Or Equal To 0?(x=w783) -> (x <= 0?=w788:bool)
        n207 = local write "State1_Time_Act"(w788) -> ()
        n208 = case shown="True" w788 {
          tunnel: w787 -> [w792 w800]
          tunnel: w786 -> [w791 w799]
          tunnel: [w792 w798] -> w785
          tunnel: [w791 w797] -> w784
          tunnel: w781 -> [_ w793]
          frame False {
          }
          frame True {
            n209 = Build Array(T2 {"Command"="Member_Release", "Data"=variant} ("State"), T2 {"Command"="Set_Interval", "Data"=variant} ("State"), w793) -> (w796:T2[])
            n210 = call-dynamic "State_FIFO.vi"("error in (no error)"=w799, "State Machine[]"=w796, "State_Machine_Class in"=w800) -> ("error out"=w797:errorcluster, "State_Machine_Class out"=w798:refnum<class "Commander.lvclass">)  [unwired: 7 in]
          }
        }
      }
      frame "Set_Time_Out" {
        n211 = call-dynamic "State_Time_Out.vi"("error in (no error)"=w804, "Parameter"=T3 {"Enable(True)"=TRUE, "Time Out_State Name"="Get_Time_Out", "Time Target (1s)"=30.0, "Time Out_Reply Message_State"="Messege_Confirm"}, "State_Machine_Class in"=w805) -> ("error out"=w802:errorcluster, "State_Machine_Class out"=w803:refnum<class "Commander.lvclass">)  [unwired: 5 in, 2 out]
      }
      frame "Get_Time_Out" {
        n212 = call-dynamic "State_Time_Out.vi"("error in (no error)"=w811, "Parameter"=T3 {"Enable(True)"=TRUE, "Time Out_State Name"="Get_Time_Out", "Time Target (1s)"=0.0, "Time Out_Reply Message_State"="Messege_Confirm"}, "State_Machine_Class in"=w812) -> ("error out"=w809:errorcluster, "Remaining Time (s)"=w808:dbl, "Timeout"=→"State1_Time_Act":bool, "State_Machine_Class out"=w810:refnum<class "Commander.lvclass">)  [unwired: 5 in]
        n213 = local write "Commander_Elapsed Time(s)"(w808) -> ()
      }
      frame "Messege_Confirm" {
        n214 = Variant To Data(error in=w815, type="", Variant=w818) -> (data=w813:string, error out=w814:errorcluster)
        n215 = One Button Dialog(message=w813) -> ()  [unwired: 1 in, 1 out]
      }
      frame "Dynamics_Release" {
        n216 = Variant To Data(error in=w825, type=refnum<class "Hyper_State_Machine.lvclass"> refnum ("SSW_Hyper_State_Machine.lvlibp:Hyper_State_Machine.lvclass"), Variant=w826) -> (data=w824:refnum<class "Hyper_State_Machine.lvclass">, error out=w823:errorcluster)
        n217 = call-dynamic "State_Lock_Unlock.vi"("error in (no error)"=w823, "Parameter"=T4 {"Action_Mode (Get)"=enum."Set", "Action_Set (False)"=FALSE, "State_In (Wait)"="Wait"}, "State_Machine_Class in"=w824) -> ("error out"=w821:errorcluster)  [unwired: 6 in, 2 out]
      }
      frame "Member_Release" {
        n218 = Build Array(w833, w832, w831, w830, w829, w828) -> (w827:refnum<class "Hyper_State_Machine.lvclass">[])
        n219 = for {
          tunnel: [w839] -> w835
          tunnel: T4 {"Action_Mode (Get)"=enum."Set", "Action_Set (False)"=FALSE, "State_In (Wait)"="Wait"} ("Parameter") -> [w838]
          tunnel: w827 -> [w837] mode=indexing
          n220 = call-dynamic "State_Lock_Unlock.vi"("Parameter"=w838, "State_Machine_Class in"=w837) -> ("error out"=w839:errorcluster)  [unwired: 7 in, 2 out]
        }
      }
      frame "Set_Wait" {
        n221 = call-dynamic "State_Lock_Unlock.vi"("error in (no error)"=w843, "Parameter"=T4 {"Action_Mode (Get)"=enum."Set", "Action_Set (False)"=TRUE, "State_In (Wait)"="Wait"}, "State_Machine_Class in"=w844) -> ("error out"=w841:errorcluster, "State_Machine_Class out"=w842:refnum<class "Commander.lvclass">)  [unwired: 6 in, 1 out]
      }
      frame "Wait" {
        n222 = call-dynamic "State_Lock_Unlock.vi"("error in (no error)"=w847, "State_Machine_Class in"=w848) -> ("error out"=w845:errorcluster, "State_Machine_Class out"=w846:refnum<class "Commander.lvclass">)  [unwired: 7 in, 1 out]
      }
      frame "Error_Action" {
        n223 = Variant To Data(error in=w849, type=w849, Variant=w852) -> (data=w851:errorcluster, error out=w850:errorcluster)
        n224 = call <vilib>:"Simple Error Handler.vi"("error in (no error)"=w851) -> ()  [unwired: 4 in, 5 out]
      }
      frame "Stop" {
        n225 = call-dynamic "State_Release.vi"("error in (no error)"=w859, "State_Machine_Class in"=w860) -> ("error out"=w857:errorcluster, "State_Machine_Class out"=w858:refnum<class "Commander.lvclass">)  [unwired: 8 in]
        n226 = call-dynamic "State_Lock_Unlock.vi"("error in (no error)"=w857, "Parameter"=T4 {"Action_Mode (Get)"=enum."Set", "Action_Set (False)"=TRUE, "State_In (Wait)"="Wait"}, "State_Machine_Class in"=w858) -> ("error out"=w855:errorcluster, "State_Machine_Class out"=w856:refnum<class "Commander.lvclass">)  [unwired: 6 in, 1 out]
      }
      frame "Exit" {
        n227 = call-dynamic "State_Release.vi"("error in (no error)"=w864, "State_Machine_Class in"=w865) -> ("error out"=w862:errorcluster, "State_Machine_Class out"=w863:refnum<class "Commander.lvclass">)  [unwired: 8 in]
      }
    }
    n228 = local read "Heart_Rate"() -> (w83:bool)
    n229 = Or(x=w178, y=w164) -> (x .or. y?=w165:bool)
    n230 = Not(x=w83) -> (.not. x?=→"Heart_Rate":bool)
    n231 = call <vilib>:"High Resolution Polling Wait.vi"("seconds to wait"="System_Wait_Time") -> ()  [unwired: 10 in, 1 out]
    n232 = call-dynamic "State_Error_Handling.vi"("error in (no error)"=w160, "Reply_State_Name"=w86, "Handling_State(State_Acquisition)"=w104, "State_Machine_Class in"=w161) -> ("error out"=w168:errorcluster)  [unwired: 6 in, 1 out]
    n233 = call-dynamic "State_Error_Handling.vi"("error in (no error)"=w145, "Reply_State_Name"=w86, "Handling_State(State_Acquisition)"=w103, "State_Machine_Class in"=w148) -> ("error out"=w141:errorcluster)  [unwired: 6 in, 1 out]
    n234 = call-dynamic "State_Error_Handling.vi"("error in (no error)"=w151, "Reply_State_Name"=w86, "Handling_State(State_Acquisition)"=w102, "State_Machine_Class in"=w152) -> ("error out"=w140:errorcluster)  [unwired: 6 in, 1 out]
    n235 = call-dynamic "State_Error_Handling.vi"("error in (no error)"=w149, "Reply_State_Name"=w86, "Handling_State(State_Acquisition)"=w101, "State_Machine_Class in"=w150) -> ("error out"=w139:errorcluster)  [unwired: 6 in, 1 out]
    n236 = call-dynamic "State_Error_Handling.vi"("error in (no error)"=w122, "Reply_State_Name"=w86, "Handling_State(State_Acquisition)"=w100, "State_Machine_Class in"=w121) -> ("error out"=w117:errorcluster)  [unwired: 6 in, 1 out]
    n237 = call-dynamic "State_Error_Handling.vi"("error in (no error)"=w88, "Reply_State_Name"=w86, "Handling_State(State_Acquisition)"=w89, "State_Machine_Class in"=w90) -> ("error out"=w87:errorcluster)  [unwired: 6 in, 1 out]
    n238 = call-dynamic "State_Error_Handling.vi"("error in (no error)"=w175, "Reply_State_Name"=w86, "Handling_State(State_Acquisition)"=w105, "State_Machine_Class in"=w106) -> ("error out"=w174:errorcluster, "State_Machine_Class out"=w173:refnum<class "Commander.lvclass">)  [unwired: 6 in]
  }
  n239 = while {
    tunnel: w24 -> [w873]
    tunnel: w23 -> [w872]
    tunnel: w22 -> [w871]
    tunnel: w21 -> [w870]
    tunnel: w20 -> [w869]
    tunnel: w19 -> [w868]
    tunnel: w18 -> [w866]
    stop <- w867 stop-if-true
    n240 = event shown="[1] \"Action Manager\": Value Change" {
      selector: _ -> [_ _ _]
      dyn-events: _ -> [_ _ _]
      timeout: _ -> [_ _ _]
      tunnel: w873 -> [_ w884 w918]
      tunnel: w872 -> [_ w883 _]
      tunnel: w871 -> [_ w882 _]
      tunnel: w870 -> [_ w881 _]
      tunnel: w869 -> [_ w880 _]
      tunnel: w868 -> [_ w879 _]
      tunnel: [_ _ TRUE] -> w867
      tunnel: w866 -> [_ w877 _]
      event Timeout {
        n241 = event-data() -> ()  [unwired: 1 in, 3 out]
      }
      event "Action Manager": Value Change {
        n242 = event-data() -> ("NewVal"=w878:T1)  [unwired: 1 in]
        n243 = Build Array(w884, w883, w882, w881, w880, w879, w877) -> (w885:refnum<class "Hyper_State_Machine.lvclass">[])
        n244 = case shown="\"Init\"" w878 {
          tunnel: w885 -> [_ w890 w898 w905 w912]
          tunnel: [w886 w888 w897 w904 w910] -> w876
          tunnel: errorcluster {"status"=FALSE, "code"=0, "source"=""} ("error out") -> [w886 w889 w896 w903 w911]
          frame "No Action", Default {
          }
          frame "Init" {
            n245 = for {
              tunnel: w890 -> [w895] mode=indexing
              shift-right: [w892] -> w888
              shift-left: w889 -> [w894]
              tunnel: T2 {"Command"="Init", "Data"=variant} ("State") -> [w891]
              n246 = call-dynamic "State_LIFO.vi"("error in (no error)"=w894, "State_Interval(Enable)"=FALSE, "State Machine"=w891, "State_Machine_Class in"=w895) -> ("error out"=w892:errorcluster)  [unwired: 6 in, 1 out]
            }
          }
          frame "Lock" {
            n247 = for {
              tunnel: w898 -> [w902] mode=indexing
              shift-right: [w900] -> w897
              shift-left: w896 -> [w899]
              n248 = call-dynamic "State_Lock_Unlock.vi"("error in (no error)"=w899, "Parameter"=T4 {"Action_Mode (Get)"=enum."Set", "Action_Set (False)"=TRUE, "State_In (Wait)"="Wait"}, "State_Machine_Class in"=w902) -> ("error out"=w900:errorcluster)  [unwired: 6 in, 2 out]
            }
          }
          frame "Unlock" {
            n249 = for {
              tunnel: w905 -> [w909] mode=indexing
              shift-right: [w907] -> w904
              shift-left: w903 -> [w906]
              n250 = call-dynamic "State_Lock_Unlock.vi"("error in (no error)"=w906, "Parameter"=T4 {"Action_Mode (Get)"=enum."Set", "Action_Set (False)"=FALSE, "State_In (Wait)"="Wait"}, "State_Machine_Class in"=w909) -> ("error out"=w907:errorcluster)  [unwired: 6 in, 2 out]
            }
          }
          frame "Release" {
            n251 = for {
              tunnel: w912 -> [w915] mode=indexing
              shift-right: [w913] -> w910
              shift-left: w911 -> [w914]
              n252 = call-dynamic "State_Release.vi"("error in (no error)"=w914, "State_Machine_Class in"=w915) -> ("error out"=w913:errorcluster)  [unwired: 8 in, 1 out]
            }
          }
        }
        n253 = property on="Action Manager" class="Enum (strict)"(error in=w876, "Blinking"=FALSE) -> ()  [unwired: 1 in, 2 out]
      }
      event "Stop": Value Change {
        n254 = event-data() -> ()  [unwired: 1 in, 6 out]
        n255 = call-dynamic "State_LIFO.vi"("State_Interval(Enable)"=FALSE, "State Machine"=T2 {"Command"="Exit", "Data"=variant} ("State"), "State_Machine_Class in"=w918) -> ()  [unwired: 7 in, 2 out]
      }
    }
  }
  n256 = call-dynamic "Get_Child_State.vi"("error in (no error)"=w16, "Hyper_State_Machine in"=w17) -> ("error out"=w15:errorcluster, "Child_State"=w13:refnum<class "State_Interface.lvclass">[], "Hyper_State_Machine out"=w14:refnum<class "Commander.lvclass">)  [unwired: 5 in, 2 out]
  n257 = Build Array (concatenate)(w14, w13) -> (w12:refnum<class "State_Interface.lvclass">[])
  n258 = for {
    tunnel: w12 -> [w925] mode=indexing
    tunnel: refnum<class "Hyper_State_Machine.lvclass"> refnum ("SSW_Hyper_State_Machine.lvlibp:Hyper_State_Machine.lvclass") -> [w924]
    shift-right: [w920] -> w10
    shift-left: w15 -> [w922]
    n259 = To More Specific Class(target class=w924, reference=w925, error in=w922) -> (specific class reference=w923:refnum<class "Hyper_State_Machine.lvclass">, error out=w921:errorcluster)
    n260 = call-dynamic "State_Destroy.vi"("error in (no error)"=w921, "State_Machine_Class in"=w923) -> ("error out"=w920:errorcluster)  [unwired: 9 in]
  }
  n261 = Merge Errors(w10, w9, w8, w7, w6, w5, w4) -> (w1:errorcluster)
  n262 = invoke class="VI" method="FP.Close"(error in=w1) -> (error out=w3:errorcluster)  [unwired: 2 in, 2 out]
  n263 = call <vilib>:"Simple Error Handler.vi"("error in (no error)"=w3) -> ("error out"=w2:errorcluster)  [unwired: 4 in, 4 out]
  n264 = disable-structure shown="RUN_TIME_ENGINE==True" {
    disable-tunnel: w2 -> [_ _]
    frame condition #0 {
      n265 = Quit LabVIEW() -> ()  [unwired: 1 in]
    }
    frame condition #1 (active) {
    }
  }
